vi "New Durability Tank Cal UI.vi"(11 "Calling VI Ref":refnum<vi>) -> ()   [LabVIEW 2019]
uses:
  Type Defs/Units Type Def (DAQ Rack).ctl
  Type Defs/New Channel Type Def (RIO).ctl
  Type Defs/Targets Type Def.ctl
  Type Defs/Target Cluster Type Def.ctl
  Type Defs/Setpoint Cluster Type Def.ctl
  Type Defs/Rack Version Type Def.ctl
  Type Defs/Registered System.ctl
  Type Defs/System Type.ctl
  Type Defs/TCP Data Stream Mode (PC).ctl
  <vilib>/Utility/miscctls.llb/LVRowAndColumnTypeDef.ctl
  <vilib>/Utility/file.llb/Write To Spreadsheet File (string).vi
  <vilib>/Utility/file.llb/Read From Spreadsheet File (string).vi
  <userlib>/_OpenG.lib/array/array.llb/Remove Duplicates from 1D Array (DBL)__ogtk.vi
  <userlib>/_OpenG.lib/array/array.llb/Search 1D Array (String)__ogtk.vi
  <vilib>/ptbypt/NI_PtbyPt.lvlib
  <vilib>/Analysis/NI_AALPro.lvlib
  <resource>/objmgr/daqmx.rc
  <vilib>/Utility/config.llb/NI_LVConfig.lvlib
  <vilib>/FTP/NI_FTP.lvlib
panel:
  out "RIO Found":bool
  out "Lost Connection":bool
  in  "Stop Second Loop":bool
  out "a0":dbl format="%#.4g"
  out "a2":dbl format="%#.4g"
  out "a1":dbl format="%#.4g"
  out "a3":dbl format="%#.4g"
  out "a4":dbl format="%#.4g"
  in  "App Dir":path
  in  "Load Indicator Tab":enum32{"Page 1"}(tab)
  in  "Header Tab":enum32{"Page 1", "Page 2"}(tab)
  in  "Header OK":bool
  in  "Header Cancel":bool
  in  "Header Comments":string[][](table)=[[""], [""], [""]]
  in  "Cal Standards Table":string[][](table)=[["", ""], ["", ""], ["", ""], ["", ""], ["", ""]]
  in  "Sys Cal Table":string[][](table)=[["", ""], ["", ""], ["", ""], ["", ""], ["", ""]]
  in  "Header Table 1":string[][](table)=[[""], [""], [""], [""], [""], [""], [""], [""]]
  in  "Header Table 2":string[][](table)=[[""], [""], [""], [""], [""], [""], [""]]
  in  "debug":bool=TRUE
  in  "Output Tab":enum32{"Page 1", "Page 2"}(tab)
  out "Row":i32
  in  "Main Tab":enum32{"Page 1", "Page 2"}(tab)
  in  "Transfer Cal":bool
  in  "Verify Tab":enum32{"Page 1", "Page 2"}(tab)
  out "Ver Reading":dbl=0.0016 caption="reading" format="%#.4g"
  in  "Hide Devs":bool
  in  "Auto":bool
  in  "Hide Cal Values":bool
  in  "Verify Edit":bool
  in  "Verify Table":string[][](table)=[["", "0", "0"], ["", "3", "3"], ["", "6", "6"], ["", "9", "9"], ["", "12", "12"], ["", "15", "15"], ["", "", ""], ["", "", ""], ["", "", ""], ["", "", ""]]
  in  "Verify Read":bool
  in  "ms":u32=1000
  in  "avg":i32=5
  in  "Save Cal":bool
  in  "Cancel Verify":bool
  in  "Cal Tab":enum32{"Apply", "Cal"}(tab)
  in  "Cancel Cal":bool
  in  "Apply Cal":bool
  in  "Confirm Cal Point":bool
  in  "Master Value":dbl caption="cal pt" format="%#.4g"
  out "Cal Reading":dbl=0.0016 caption="reading" format="%#.4g"
  in  "Channel to Cal":T1
  in  "4th Point Cal":bool
  out "Reading Value 4":dbl caption="reading" format="%#.4g"
  in  "Cal Value 4":dbl caption="cal pt" format="%#.4g"
  in  "5th Point Cal":bool
  out "Reading Value 5":dbl caption="reading" format="%#.4g"
  in  "Cal Value 5":dbl caption="cal pt" format="%#.4g"
  in  "Start Verification":bool
  in  "Header":bool
  out "Cal Table":string[][](table)=[["AI-00", "V", "", "", "", "", "", "", "", "", "", "", "", "", "", "", "", "", "", "", "", "", "", "", "", "", "", "", "", "", "", ""], ["AI-01", "V", "", "", "", "", "", "", "", "", "", "", "", "", "", "", "", "", "", "", "", "", "", "", "", "", "", "", "", "", "", ""], ["AI-02", "V", "", "", "", "", "", "", "", "", "", "", "", "", "", "", "", "", "", "", "", "", "", "", "", "", "", "", "", "", "", ""], ["AI-03", "V", "", "", "", "", "", "", "", "", "", "", "", "", "", "", "", "", "", "", "", "", "", "", "", "", "", "", "", "", "", ""], ["AI-04", "V", "", "", "", "", "", "", "", "", "", "", "", "", "", "", "", "", "", "", "", "", "", "", "", "", "", "", "", "", "", ""], ["AI-05", "V", "", "", "", "", "", "", "", "", "", "", "", "", "", "", "", "", "", "", "", "", "", "", "", "", "", "", "", "", "", ""], ["AI-06", "V", "", "", "", "", "", "", "", "", "", "", "", "", "", "", "", "", "", "", "", "", "", "", "", "", "", "", "", "", "", ""], ["AI-07", "V", "", "", "", "", "", "", "", "", "", "", "", "", "", "", "", "", "", "", "", "", "", "", "", "", "", "", "", "", "", ""], ["AI-08", "V", "", "", "", "", "", "", "", "", "", "", "", "", "", "", "", "", "", "", "", "", "", "", "", "", "", "", "", "", "", ""], ["AI-09", "V", "", "", "", "", "", "", "", "", "", "", "", "", "", "", "", "", "", "", "", "", "", "", "", "", "", "", "", "", "", ""], ["AI-10", "V", "", "", "", "", "", "", "", "", "", "", "", "", "", "", "", "", "", "", "", "", "", "", "", "", "", "", "", "", "", ""], ["AI-11", "V", "", "", "", "", "", "", "", "", "", "", "", "", "", "", "", "", "", "", "", "", "", "", "", "", "", "", "", "", "", ""], ["AI-12", "V", "", "", "", "", "", "", "", "", "", "", "", "", "", "", "", "", "", "", "", "", "", "", "", "", "", "", "", "", "", ""], ["AI-13", "V", "", "", "", "", "", "", "", "", "", "", "", "", "", "", "", "", "", "", "", "", "", "", "", "", "", "", "", "", "", ""], ["AI-14", "V", "", "", "", "", "", "", "", "", "", "", "", "", "", "", "", "", "", "", "", "", "", "", "", "", "", "", "", "", "", ""], ["AI-15", "V", "", "", "", "", "", "", "", "", "", "", "", "", "", "", "", "", "", "", "", "", "", "", "", "", "", "", "", "", "", ""], ["AI-16", "V", "", "", "", "", "", "", "", "", "", "", "", "", "", "", "", "", "", "", "", "", "", "", "", "", "", "", "", "", "", ""], ["AI-17", "V", "", "", "", "", "", "", "", "", "", "", "", "", "", "", "", "", "", "", "", "", "", "", "", "", "", "", "", "", "", ""], ["AI-18", "V", "", "", "", "", "", "", "", "", "", "", "", "", "", "", "", "", "", "", "", "", "", "", "", "", "", "", "", "", "", ""], ["AI-19", "V", "", "", "", "", "", "", "", "", "", "", "", "", "", "", "", "", "", "", "", "", "", "", "", "", "", "", "", "", "", ""], ["AI-20", "V", "", "", "", "", "", "", "", "", "", "", "", "", "", "", "", "", "", "", "", "", "", "", "", "", "", "", "", "", "", ""], ["AI-21", "V", "", "", "", "", "", "", "", "", "", "", "", "", "", "", "", "", "", "", "", "", "", "", "", "", "", "", "", "", "", ""], ["AI-22", "V", "", "", "", "", "", "", "", "", "", "", "", "", "", "", "", "", "", "", "", "", "", "", "", "", "", "", "", "", "", ""], ["AI-23", "V", "", "", "", "", "", "", "", "", "", "", "", "", "", "", "", "", "", "", "", "", "", "", "", "", "", "", "", "", "", ""], ["AI-24", "V", "", "", "", "", "", "", "", "", "", "", "", "", "", "", "", "", "", "", "", "", "", "", "", "", "", "", "", "", "", ""], ["AI-25", "V", "", "", "", "", "", "", "", "", "", "", "", "", "", "", "", "", "", "", "", "", "", "", "", "", "", "", "", "", "", ""], ["AI-26", "V", "", "", "", "", "", "", "", "", "", "", "", "", "", "", "", "", "", "", "", "", "", "", "", "", "", "", "", "", "", ""], ["AI-27", "V", "", "", "", "", "", "", "", "", "", "", "", "", "", "", "", "", "", "", "", "", "", "", "", "", "", "", "", "", "", ""], ["AI-28", "V", "", "", "", "", "", "", "", "", "", "", "", "", "", "", "", "", "", "", "", "", "", "", "", "", "", "", "", "", "", ""], ["AI-29", "V", "", "", "", "", "", "", "", "", "", "", "", "", "", "", "", "", "", "", "", "", "", "", "", "", "", "", "", "", "", ""], ["AI-30", "V", "", "", "", "", "", "", "", "", "", "", "", "", "", "", "", "", "", "", "", "", "", "", "", "", "", "", "", "", "", ""], ["AI-31", "V", "", "", "", "", "", "", "", "", "", "", "", "", "", "", "", "", "", "", "", "", "", "", "", "", "", "", "", "", "", ""], ["TC-00", "degF", "", "", "", "", "", "", "", "", "", "", "", "", "", "", "", "", "", "", "", "", "", "", "", "", "", "", "", "", "", ""], ["TC-01", "degF", "", "", "", "", "", "", "", "", "", "", "", "", "", "", "", "", "", "", "", "", "", "", "", "", "", "", "", "", "", ""], ["TC-02", "degF", "", "", "", "", "", "", "", "", "", "", "", "", "", "", "", "", "", "", "", "", "", "", "", "", "", "", "", "", "", ""], ["TC-03", "degF", "", "", "", "", "", "", "", "", "", "", "", "", "", "", "", "", "", "", "", "", "", "", "", "", "", "", "", "", "", ""], ["TC-04", "degF", "", "", "", "", "", "", "", "", "", "", "", "", "", "", "", "", "", "", "", "", "", "", "", "", "", "", "", "", "", ""], ["TC-05", "degF", "", "", "", "", "", "", "", "", "", "", "", "", "", "", "", "", "", "", "", "", "", "", "", "", "", "", "", "", "", ""], ["TC-06", "degF", "", "", "", "", "", "", "", "", "", "", "", "", "", "", "", "", "", "", "", "", "", "", "", "", "", "", "", "", "", ""], ["TC-07", "degF", "", "", "", "", "", "", "", "", "", "", "", "", "", "", "", "", "", "", "", "", "", "", "", "", "", "", "", "", "", ""], ["TC-08", "degF", "", "", "", "", "", "", "", "", "", "", "", "", "", "", "", "", "", "", "", "", "", "", "", "", "", "", "", "", "", ""], ["TC-09", "degF", "", "", "", "", "", "", "", "", "", "", "", "", "", "", "", "", "", "", "", "", "", "", "", "", "", "", "", "", "", ""], ["TC-10", "degF", "", "", "", "", "", "", "", "", "", "", "", "", "", "", "", "", "", "", "", "", "", "", "", "", "", "", "", "", "", ""], ["TC-11", "degF", "", "", "", "", "", "", "", "", "", "", "", "", "", "", "", "", "", "", "", "", "", "", "", "", "", "", "", "", "", ""], ["TC-12", "degF", "", "", "", "", "", "", "", "", "", "", "", "", "", "", "", "", "", "", "", "", "", "", "", "", "", "", "", "", "", ""], ["TC-13", "degF", "", "", "", "", "", "", "", "", "", "", "", "", "", "", "", "", "", "", "", "", "", "", "", "", "", "", "", "", "", ""], ["TC-14", "degF", "", "", "", "", "", "", "", "", "", "", "", "", "", "", "", "", "", "", "", "", "", "", "", "", "", "", "", "", "", ""], ["TC-15", "degF", "", "", "", "", "", "", "", "", "", "", "", "", "", "", "", "", "", "", "", "", "", "", "", "", "", "", "", "", "", ""], ["", "", "", "", "", "", "", "", "", "", "", "", "", "", "", "", "", "", "", "", "", "", "", "", "", "", "", "", "", "", "", ""]]
  out "Tank IP:":string
  in  "Start Cal":bool
  in  "1st Point Cal":bool
  out "Reading Value 1":dbl caption="Read Data" format="%#.4g"
  in  "Cal Value 1":dbl caption="Cal Point" format="%#.4g"
  in  "2nd Point Cal":bool
  out "Reading Value 2":dbl caption="reading" format="%#.4g"
  in  "Cal Value 2":dbl caption="cal pt" format="%#.4g"
  in  "Cal Unit":T2
  in  "3rd Point Cal":bool
  out "Reading Value 3":dbl caption="reading" format="%#.4g"
  in  "Cal Value 3":dbl caption="cal pt" format="%#.4g"
  in  "View Spreadsheet":bool
  # "Channel Data"
  # "System Calibration Components"
  # "Calibration Standards Used"
  # "Output Control"
  # "Enter Header Info"
  # "Calibration"
  # "Verification"
  # "Select Channel to Calibrate"
  # "Cal Spreadsheet"
  # "*Excel must be closed to return control to this app."
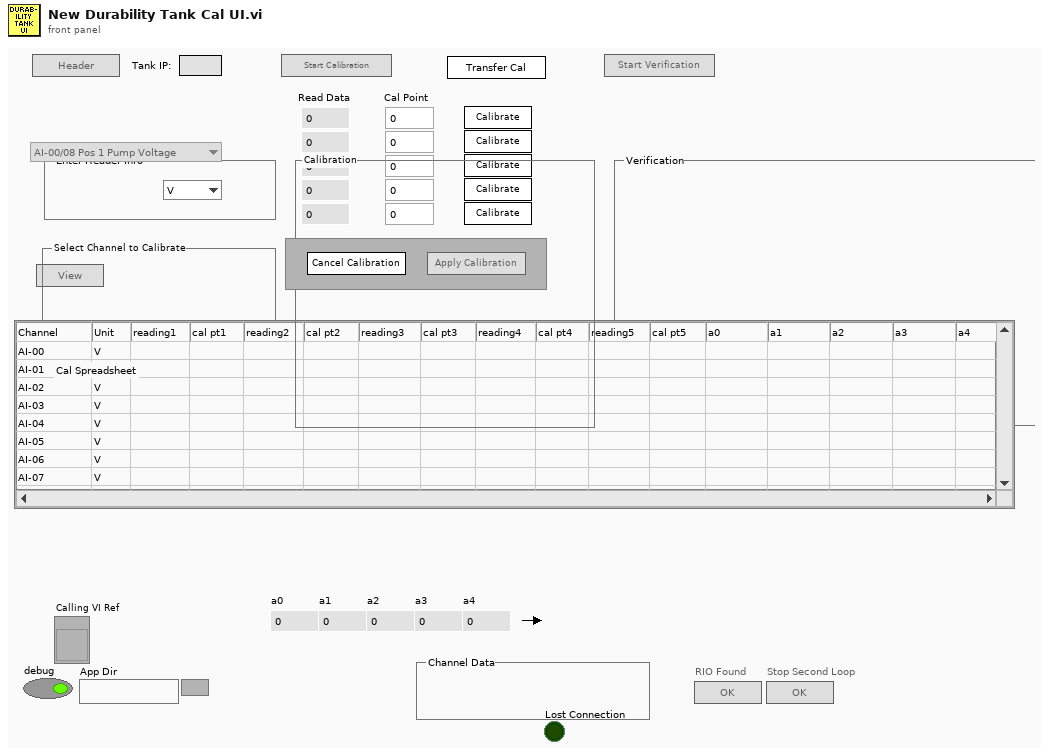
[diagram p1: front panel]
types:
  T1 = typedef "New Channel Type Def (RIO).ctl" = enum16{"AI-00/08 Pos 1 Pump Voltage", "AI-01/09 Pos 2 Pump Voltage", "AI-02/10 Pos 3 Pump Voltage", "AI-03/11 Pos 4 Pump Voltage", "AI-04/12 Pos 5 Pump Voltage", "AI-05/13 Pos 6 Pump Voltage", "AI-06 Spare", "AI-14 Spare", "AI-07 Spare", "AI-15 Power Supply Voltage", "AI-16 Pos 1 Pump Current", "AI-17 Pos 2 Pump Current", "AI-18 Pos 3 Pump Current", "AI-19 Pos 4 Pump Current", "AI-20 Pos 5 Pump Current", "AI-21 Pos 6 Pump Current", "AI-16 Pos 1 Pump Speed", "AI-17 Pos 2 Pump Speed", "AI-18 Pos 3 Pump Speed", "AI-19 Pos 4 Pump Speed", "AI-20 Pos 5 Pump Speed", "AI-21 Pos 6 Pump Speed", "AI-22 Pos 1 Controller Current", "AI-23 Pos 2 Controller Current", "AI-24 Pos 3 Controller Current", "AI-25 Pos 4 Controller Current", "AI-26 Pos 5 Controller Current", "AI-27 Pos 6 Controller Current", "AI-28 Tank 1 Temperature", "AI-29 Tank 2 Temperature", "AI-30 Pos 1 Pump Pressure", "AI-31 Pos 2 Pump Pressure", "AI-32 Pos 3 Pump Pressure", "AI-33 Pos 4 Pump Pressure", "AI-34 Pos 5 Pump Pressure", "AI-35 Pos 6 Pump Pressure", "AI-36 Pos 1 Pump Flow", "AI-37 Pos 2 Pump Flow", "AI-38 Pos 3 Pump Flow", "AI-39 Pos 4 Pump Flow", "AI-40 Pos 5 Pump Flow", "AI-41 Pos 6 Pump Flow", "AI-42 Spare", "AI-43 Spare", "AI-44 Spare", "AI-45 Spare", "AI-46 Spare", "AI-47 Spare", "AI-00/08 Pos 1 Controller Voltage", "AI-01/09 Pos 2 Controller Voltage", "AI-02/10 Pos 3 Controller Voltage", "AI-03/11 Pos 4 Controller Voltage", "AI-04/12 Pos 5 Controller Voltage", "AI-05/13 Pos 6 Controller Voltage"}
  T2 = typedef "Units Type Def (DAQ Rack).ctl" = enum16{"V", "mA", "A", "Hz", "deg C"}
  T3 = typedef "Registered System.ctl" = cluster{"System Type":T4, "Serial Number":u32, "ID":string, "Cal File?":bool}
  T4 = typedef "System Type.ctl" = enum16{"DAQ Rack", "DAQ Cart", "RIO", "unknown", "open"}
  T5 = typedef "Rack Version Type Def.ctl" = enum16{"Volts & TC", "Volts", "RIO", "Volts & Current", "Cart"}
  T6 = typedef "Targets Type Def.ctl" = cluster{"V Targets":T7, "5V Targets":T7, "mA Targets":T7, "A Targets":T7, "Hz Targets":T7, "TC Targets":T7, "V Setpoints":T8, "5V Setpoints":T8, "mA Setpoints ":T8, "A Setpoints":T8, "Hz Setpoints":T8, "25A Setpoints":T8, "25A Targets":T7, "CT Targets":T7, "DegC Targets":T7, "kPa Targets":T7, "LpH Targets":T7, "CT Setpoints":T8, "DegC Setpoints":T8, "kPa Setpoints":T8, "LpH Setpoints":T8}
  T7 = typedef "Target Cluster Type Def.ctl" = cluster{"target1":dbl, "target2":dbl, "target3":dbl, "target4":dbl, "target5":dbl, "target6":dbl, "target7":dbl, "target8":dbl, "target9":dbl, "target10":dbl}
  T8 = typedef "Setpoint Cluster Type Def.ctl" = cluster{"setpoint1":dbl, "setpoint2":dbl, "setpoint3":dbl, "setpoint4":dbl, "setpoint5":dbl}
  T9 = cluster{"Error":errorcluster, "Cal Log":string[][], "Cal Log Header":string[], "Cal Files Base Path":path, "Default Cal Log":string[][], "Samples to Avg":i32, "Base Path":path, "Cal Targets Path":path, "Calling VI Ref":refnum<vi>, "Selected Chassis":tag, "debug":bool, "Verify Table":string[][], "Cal Template Path":path, "Cal Spreadsheet Path":path, "Verify Table Ref":refnum<vi>, "Init Mean":bool, "Auto":bool, "App Dir":path, "DAQ Rack":string, "Cal File Path":path, "Targets":T6, "Cal Unit":T2, "Channel to Cal":T1, "Rack Version":T5, "Verification":bool, "Registered Systems":T3[], "Desired System":T3, "Cal Target Array":string[], "LastCalPt":i32, "StreamCtrlActive":bool}
  T10 = enum8{"Enabled", "Disabled", "Disabled and Grayed Out"}
  T11 = typedef "TCP Data Stream Mode (PC).ctl" = enum16{"Init", "Read Data", "Close"}
  T12 = typedef "LVRowAndColumnTypeDef.ctl" = cluster{"Row":i32, "Column":i32}
  T13 = enum32{"Bad", "Idle", "Run top level", "Running"}
  T14 = cluster{"[0]":dbl, "[1]":dbl, "[2]":dbl, "[3]":dbl, "[4]":dbl, "[5]":dbl, "[6]":dbl, "[7]":dbl, "[8]":dbl, "[9]":dbl}
  T15 = typedef "NI_LVConfig.lvlib/Config Data RefNum.ctl" = refnum<k1>
  T16 = cluster{"Error":errorcluster, "Cal Log":string[][], "Cal Log Header":string[], "Cal Files Base Path":path, "Default Cal Log":string[][], "Samples to Avg":i32, "Base Path":path, "Cal Targets Path":path, "Calling VI Ref":refnum<vi>, "Selected Chassis":tag, "debug":bool, "Verify Table":string[][], "Cal Template Path":path, "Cal Spreadsheet Path":path, "Verify Table Ref":refnum<vi>, "Init Mean":bool, "Auto":bool, "App Dir":path, "DAQ Rack":string, "Cal File Path":path, "Targets":T6, "Cal Unit":T2, "Channel to Cal":T1, "Rack Version":T5, "Verification":bool, "Registered Systems":T3[], "Desired System":T3, "Cal Target Array":string[], "LastCalPt":i32}
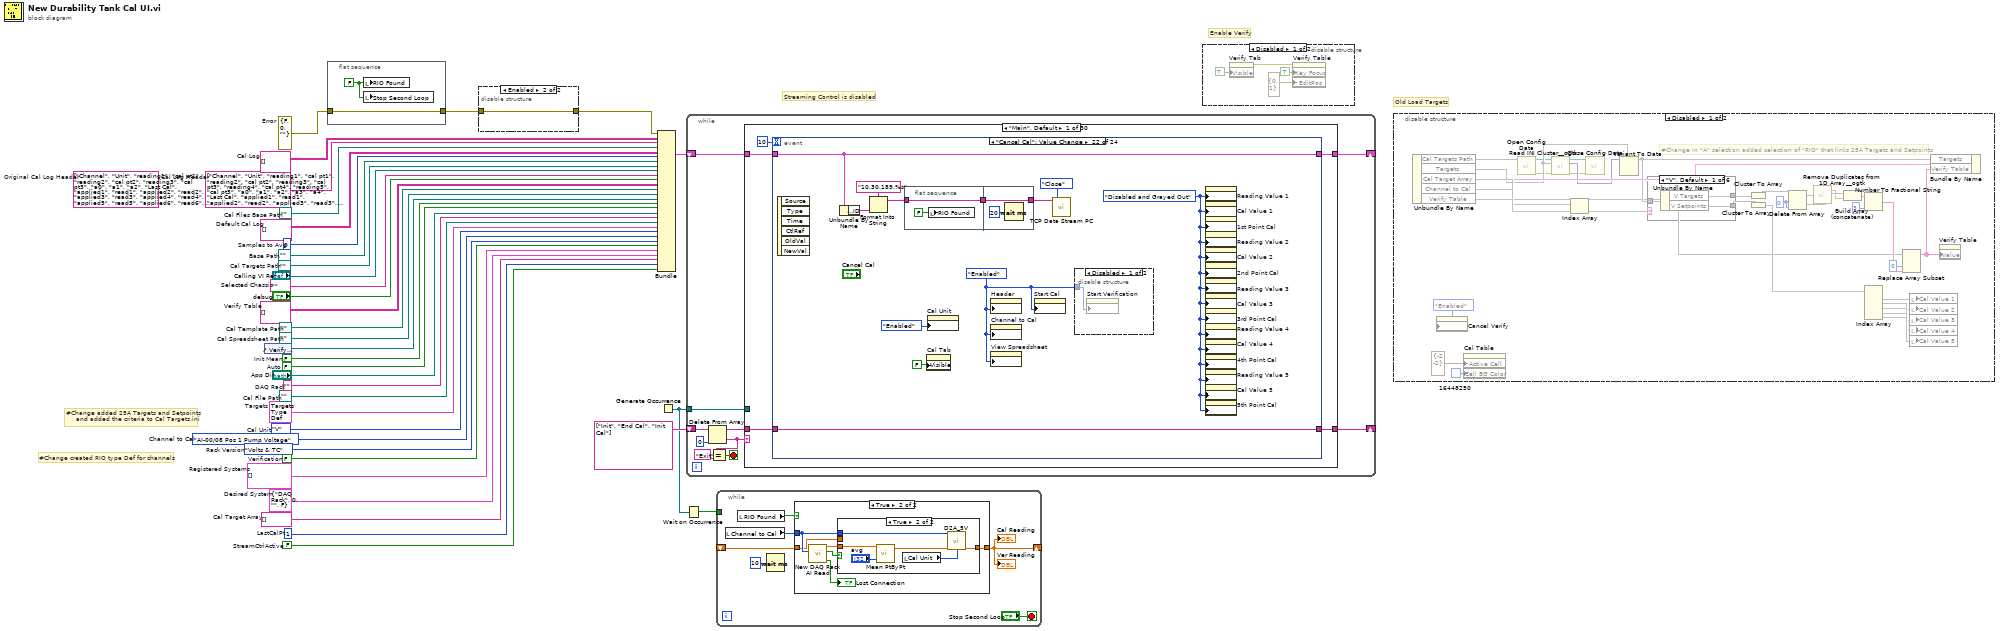
[diagram p0: block diagram]
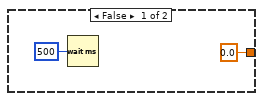
[diagram p2: hidden frame]
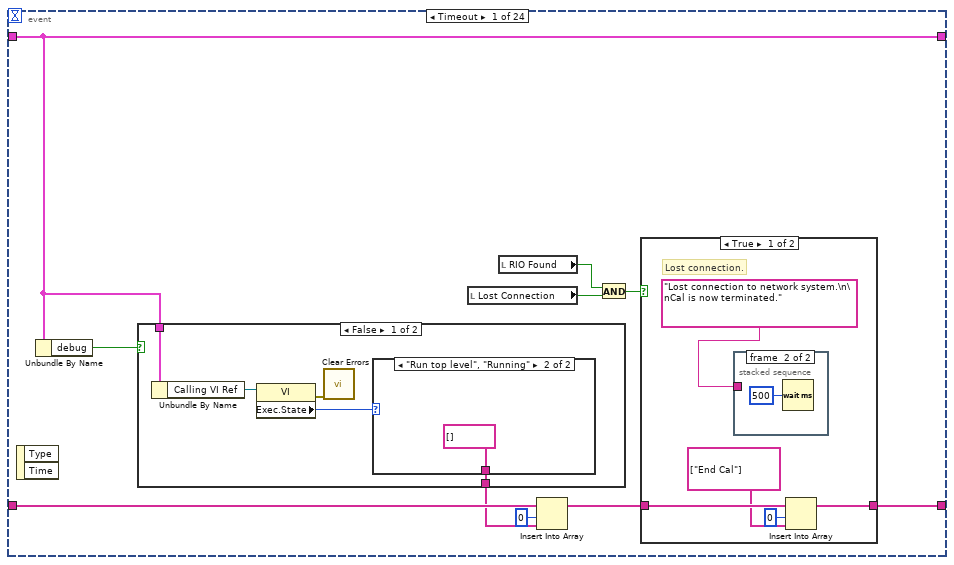
[diagram p4: hidden frame]
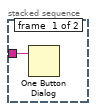
[diagram p5: hidden frame]
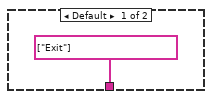
[diagram p7: hidden frame]
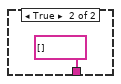
[diagram p8: hidden frame]
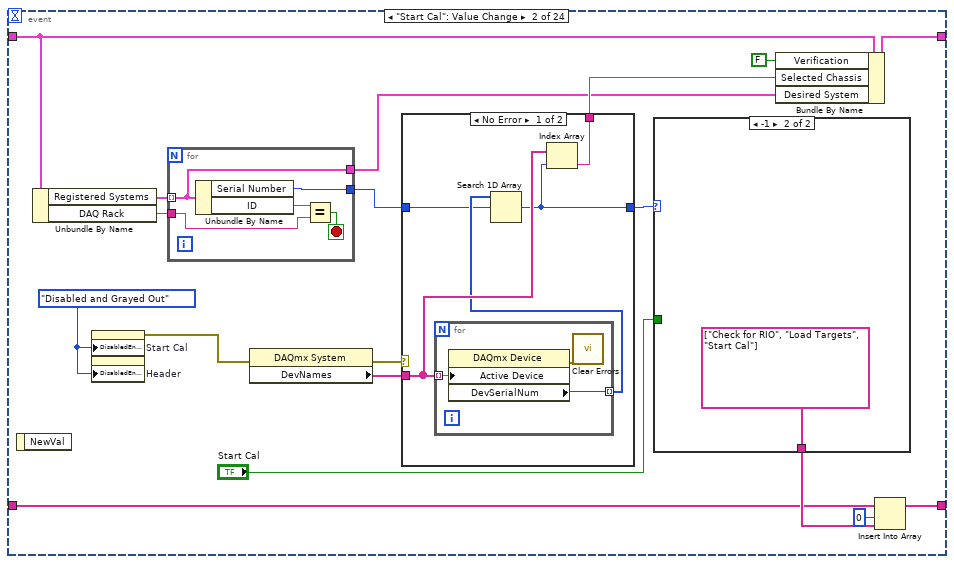
[diagram p9: hidden frame]
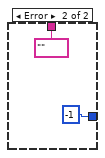
[diagram p10: hidden frame]
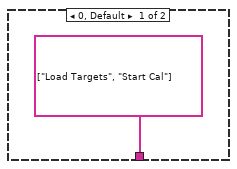
[diagram p11: hidden frame]
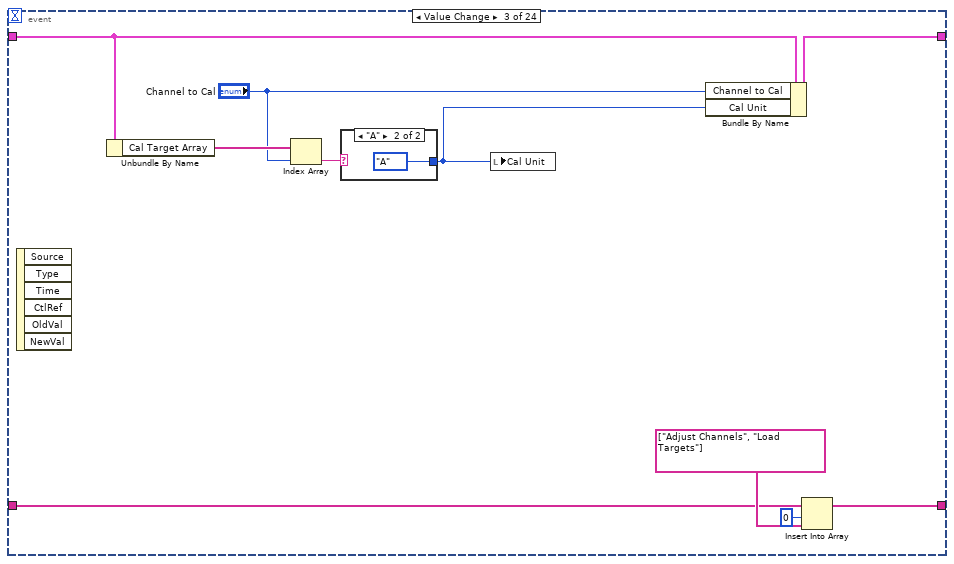
[diagram p12: hidden frame]
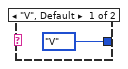
[diagram p13: hidden frame]
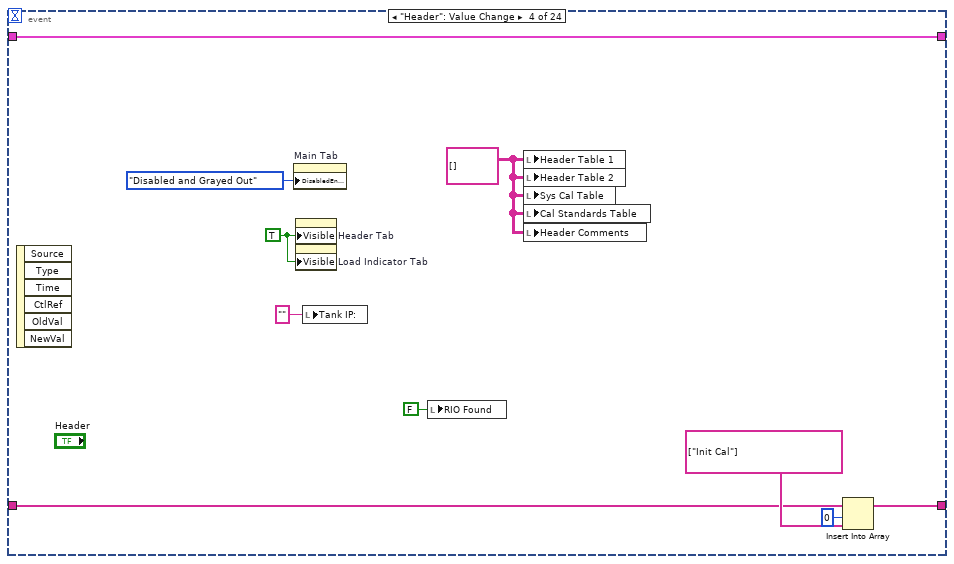
[diagram p14: hidden frame]
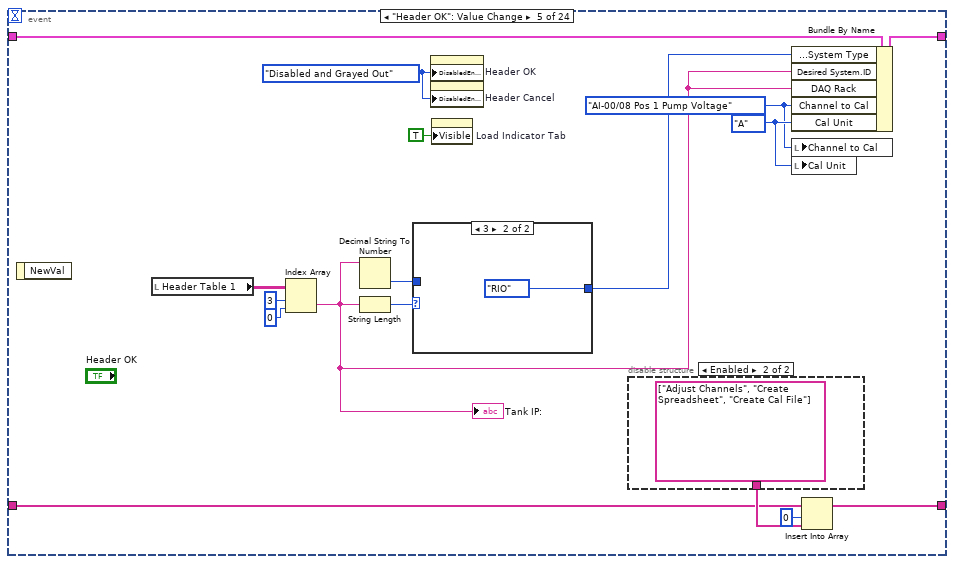
[diagram p15: hidden frame]
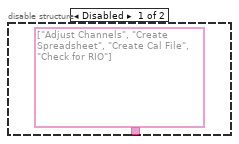
[diagram p16: hidden frame]
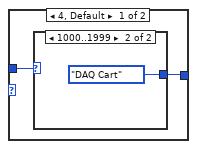
[diagram p17: hidden frame]
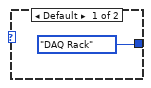
[diagram p18: hidden frame]
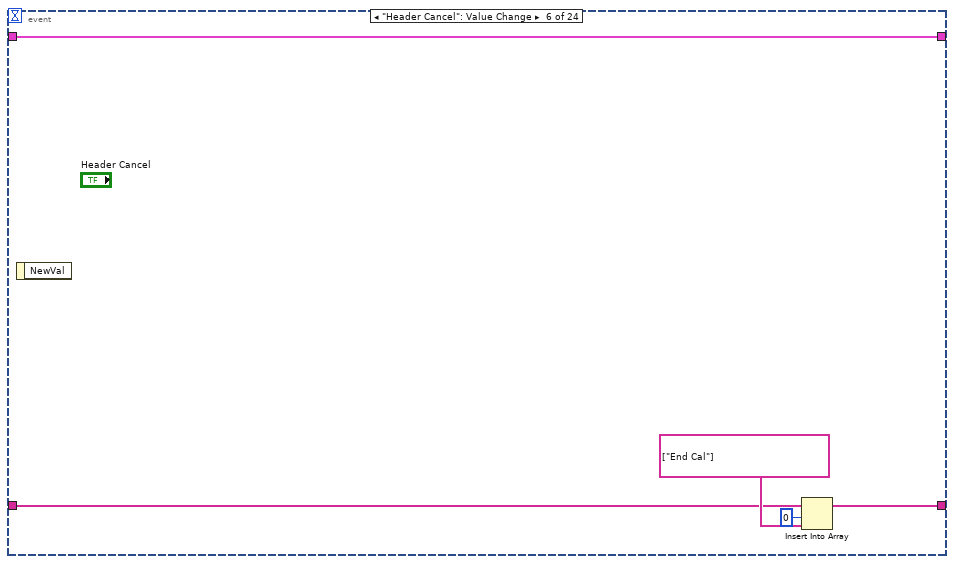
[diagram p19: hidden frame]
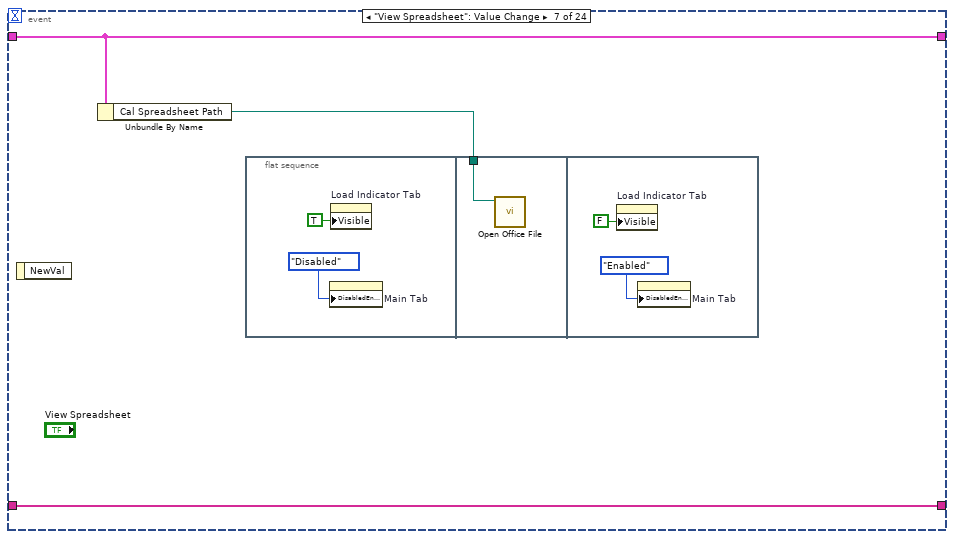
[diagram p20: hidden frame]
diagram:
  w7 = FALSE  # StreamCtrlActive
  w8 = 1  # LastCalPt
  w10 = New_Channel_Type_Def_(RIO)."AI-00/08 Pos 1 Pump Voltage"  # Channel to Cal
  w11 = string[] ["Channel", "Unit", "reading1", "cal pt1", "reading2", "cal pt2", "reading3", "cal pt3", "reading4", "cal pt4", "reading5", "cal pt5", "a0", "a1", "a2", "a3", "a4", "Last Cal", "applied1", "read1", "applied2", "read2", "applied3", "read3", "applied4", "read4", "applied5", "read5", "applied6", "read6", "applied7", "read7", "applied8", "read8", "applied9", "read9", "applied10", "read10"]  # Cal Log Header
  w12 = string[] []  # Cal Target Array
  w13 = T3 {"System Type"=enum."DAQ Rack", "Serial Number"=0, "ID"="", "Cal File?"=FALSE}  # Desired System
  w14 = T3[] []  # Registered Systems
  w15 = FALSE  # Verification
  w16 = Rack_Version_Type_Def."Volts & TC"  # Rack Version
  w17 = Units_Type_Def_(DAQ_Rack)."V"  # Cal Unit
  w18 = T6 {"V Targets"={"target1"=0.0, "target2"=0.0, "target3"=0.0, "target4"=0.0, "target5"=0.0, "target6"=0.0, "target7"=0.0, "target8"=0.0, "target9"=0.0, "target10"=0.0}, "5V Targets"={"target1"=0.0, "target2"=0.0, "target3"=0.0, "target4"=0.0, "target5"=0.0, "target6"=0.0, "target7"=0.0, "target8"=0.0, "target9"=0.0, "target10"=0.0}, "mA Targets"={"target1"=0.0, "target2"=0.0, "target3"=0.0, "target4"=0.0, "target5"=0.0, "target6"=0.0, "target7"=0.0, "target8"=0.0, "target9"=1.0, "target10"=0.0}, "A Targets"={"target1"=0.0, "target2"=0.0, "target3"=0.0, "target4"=0.0, "target5"=0.0, "target6"=0.0, "target7"=0.0, "target8"=0.0, "target9"=0.0, "target10"=0.0}, "Hz Targets"={"target1"=0.0, "target2"=0.0, "target3"=0.0, "target4"=0.0, "target5"=0.0, "target6"=0.0, "target7"=0.0, "target8"=0.0, "target9"=0.0, "target10"=0.0}, "TC Targets"={"target1"=0.0, "target2"=0.0, "target3"=0.0, "target4"=0.0, "target5"=0.0, "target6"=0.0, "target7"=0.0, "target8"=0.0, "target9"=0.0, "target10"=0.0}, "V Setpoints"={"setpoint1"=0.0, "setpoint2"=0.0, "setpoint3"=0.0, "setpoint4"=0.0, "setpoint5"=0.0}, "5V Setpoints"={"setpoint1"=0.0, "setpoint2"=0.0, "setpoint3"=0.0, "setpoint4"=0.0, "setpoint5"=0.0}, "mA Setpoints "={"setpoint1"=0.0, "setpoint2"=0.0, "setpoint3"=0.0, "setpoint4"=0.0, "setpoint5"=0.0}, "A Setpoints"={"setpoint1"=0.0, "setpoint2"=0.0, "setpoint3"=0.0, "setpoint4"=0.0, "setpoint5"=0.0}, "Hz Setpoints"={"setpoint1"=0.0, "setpoint2"=0.0, "setpoint3"=0.0, "setpoint4"=0.0, "setpoint5"=0.0}, "25A Setpoints"={"setpoint1"=0.0, "setpoint2"=0.0, "setpoint3"=0.0, "setpoint4"=0.0, "setpoint5"=0.0}, "25A Targets"={"target1"=0.0, "target2"=0.0, "target3"=0.0, "target4"=0.0, "target5"=0.0, "target6"=0.0, "target7"=0.0, "target8"=0.0, "target9"=0.0, "target10"=0.0}, "CT Targets"={"target1"=0.0, "target2"=0.0, "target3"=0.0, "target4"=0.0, "target5"=0.0, "target6"=0.0, "target7"=0.0, "target8"=0.0, "target9"=0.0, "target10"=0.0}, "DegC Targets"={"target1"=0.0, "target2"=0.0, "target3"=0.0, "target4"=0.0, "target5"=0.0, "target6"=0.0, "target7"=0.0, "target8"=0.0, "target9"=0.0, "target10"=0.0}, "kPa Targets"={"target1"=0.0, "target2"=0.0, "target3"=0.0, "target4"=0.0, "target5"=0.0, "target6"=0.0, "target7"=0.0, "target8"=0.0, "target9"=0.0, "target10"=0.0}, "LpH Targets"={"target1"=0.0, "target2"=0.0, "target3"=0.0, "target4"=0.0, "target5"=0.0, "target6"=0.0, "target7"=0.0, "target8"=0.0, "target9"=0.0, "target10"=0.0}, "CT Setpoints"={"setpoint1"=0.0, "setpoint2"=0.0, "setpoint3"=0.0, "setpoint4"=0.0, "setpoint5"=0.0}, "DegC Setpoints"={"setpoint1"=0.0, "setpoint2"=0.0, "setpoint3"=0.0, "setpoint4"=0.0, "setpoint5"=0.0}, "kPa Setpoints"={"setpoint1"=0.0, "setpoint2"=0.0, "setpoint3"=0.0, "setpoint4"=0.0, "setpoint5"=0.0}, "LpH Setpoints"={"setpoint1"=0.0, "setpoint2"=0.0, "setpoint3"=0.0, "setpoint4"=0.0, "setpoint5"=0.0}}  # Targets
  w19 = path ""  # Cal File Path
  w20 = ""  # DAQ Rack
  w22 = FALSE  # Auto
  w23 = FALSE  # Init Mean
  w25 = path ""  # Cal Spreadsheet Path
  w26 = path ""  # Cal Template Path
  w27 = string[][] []  # Verify Table
  w29 = tag ""  # Selected Chassis
  w31 = path ""  # Cal Targets Path
  w32 = path ""  # Base Path
  w33 = 0  # Samples to Avg
  w34 = string[][] []  # Default Cal Log
  w35 = path ""  # Cal Files Base Path
  (unwired) string[] ["Channel", "Unit", "reading1", "cal pt1", "reading2", "cal pt2", "reading3", "cal pt3", "a0", "a1", "a2", "Last Cal", "applied1", "read1", "applied2", "read2", "applied3", "read3", "applied4", "read4", "applied5", "read5", "applied6", "read6", "applied7", "read7", "applied8", "read8", "applied9", "read9", "applied10", "read10"]  # Original Cal Log Header
  w36 = string[][] []  # Cal Log
  w9 = errorcluster {"status"=FALSE, "code"=0, "source"=""}  # Error
  # "Old Load Targets"
  # "Streaming Control is disabled"
  # "Enable Verify"
  # "#Change created RIO type Def for channels"
  # "#Change added 25A Targets and Setpoints\n     and added the criteria to Cal Targets.ini"
  n1 = control-ref of="Verify Table Ref"() -> (w24:refnum<vi>)
  n2 = flat-sequence {
    tunnel: w9 -> [w38]
    tunnel: [w38] -> w6
    frame #0 {
      w37 = FALSE ("RIO Found")
      n3 = local write "RIO Found"(w37) -> ()
      n4 = local write "Stop Second Loop"(w37) -> ()
    }
  }
  n5 = disable-structure shown="Enabled" {
    disable-tunnel: w6 -> [w42 w43]
    disable-tunnel: [w40 w43] -> w5
    frame Disabled {
      w39 = TRUE ("Visible")
      n6 = property on="Cal Tab" class="TabCtl (strict)"(error in=w42, "Visible"=w39) -> (error out=w41:errorcluster)  [unwired: 1 in, 1 out]
      n7 = property on="Verify Tab" class="TabCtl (strict)"(error in=w41, "Visible"=w39) -> (error out=w40:errorcluster)  [unwired: 1 in, 1 out]
    }
    frame Enabled {
    }
  }
  n8 = Bundle("Error"=w5, "Cal Log"=w36, "Cal Log Header"=w11, "Cal Files Base Path"=w35, "Default Cal Log"=w34, "Samples to Avg"=w33, "Base Path"=w32, "Cal Targets Path"=w31, "Calling VI Ref"="Calling VI Ref", "Selected Chassis"=w29, "debug"="debug", "Verify Table"=w27, "Cal Template Path"=w26, "Cal Spreadsheet Path"=w25, "Verify Table Ref"=w24, "Init Mean"=w23, "Auto"=w22, "App Dir"="App Dir", "DAQ Rack"=w20, "Cal File Path"=w19, "Targets"=w18, "Cal Unit"=w17, "Channel to Cal"=w10, "Rack Version"=w16, "Verification"=w15, "Registered Systems"=w14, "Desired System"=w13, "Cal Target Array"=w12, "LastCalPt"=w8, "StreamCtrlActive"=w7) -> (w3:T9)  [unwired: 1 in]
  n9 = Generate Occurrence() -> (w2:refnum<k4>)
  n10 = Wait on Occurrence(2:w2) -> (0:w1:bool)  [unwired: 2 in]
  n11 = while {
    shift-right: [w46] -> _
    shift-left: string[] ["Init", "End Cal", "Init Cal"] -> [w53]
    shift-right: [w48] -> _
    shift-left: w3 -> [w49]
    tunnel: w2 -> [w44]
    stop <- w52 stop-if-true
    n12 = Delete From Array(array=w53, index=0) -> (deleted portion=w45:string, array with subset deleted=w51:string[])  [unwired: 1 in]
    n13 = Equal?(x=w45, y="Exit" ("x")) -> (x = y?=w52:bool)
    n14 = case shown="\"Main\", Default" w45 {
      selector: w45 -> [_ _ _ _ _ _ _ _ _ _ _ _ _ _ _ w851 _ _ _ _ _ _ _ _ _ _ _ _ _ _]
      tunnel: w51 -> [w57 w425 w440 w448 w464 w513 w543 w546 w550 w581 w610 w639 w663 w721 w840 w853 w867 w883 w967 w994 w1004 w1067 w1145 w1168 w1185 w1196 w1219 w1232 w1240 w1243]
      tunnel: w49 -> [w56 w418 w441 w454 w461 w512 w542 w545 w548 w584 w612 w633 w661 w769 w844 w848 w868 w877 w953 w978 w1005 w1028 w1106 w1167 w1183 w1194 w1216 w1229 w1238 w1242]
      tunnel: [w55 w400 w441 w453 w461 w511 w541 w545 w548 w583 w612 w632 w665 w778 w844 w847 w868 w877 w953 w973 w1005 w1028 w1106 w1167 w1182 w1194 w1216 w1229 w1239 w1242] -> w48
      tunnel: [w54 w425 w440 w445 w463 w513 w543 w546 w549 w582 w611 w640 w664 w720 w840 w853 w867 w884 w966 w995 w1004 w1068 w1146 w1168 w1184 w1195 w1219 w1233 w1240 w1243] -> w46
      tunnel: w44 -> [_ w399 _ _ _ _ _ _ _ _ _ _ _ _ _ _ _ _ _ _ _ _ _ _ _ _ _ _ _ _]
      frame "Main", Default {
        n15 = event shown="[21] \"Cancel Cal\": Value Change" {
          selector: _ -> [_ _ _ _ _ _ _ _ _ _ _ _ _ _ _ _ _ _ _ _ _ _ _ _]
          dyn-events: _ -> [_ _ _ _ _ _ _ _ _ _ _ _ _ _ _ _ _ _ _ _ _ _ _ _]
          timeout: 10 -> [_ _ _ _ _ _ _ _ _ _ _ _ _ _ _ _ _ _ _ _ _ _ _ _]
          tunnel: w57 -> [w68 w100 w126 w136 w154 w169 w173 _ _ _ _ _ _ w232 w257 _ w300 _ w319 w352 w358 w381 w389 w395]
          tunnel: [w66 w96 w129 w141 w148 w167 w171 w186 w194 w202 w210 w218 w221 w235 w259 w294 w298 w307 w320 w353 w356 w374 w391 w396] -> w55
          tunnel: w56 -> [w66 w97 w124 w141 w149 w167 w171 w186 w194 w202 w210 w218 w221 w237 w259 w294 w299 w308 w320 w353 w356 w374 w391 w397]
          tunnel: [w61 w101 w125 w135 w155 w168 w173 w183 w191 w199 w207 w215 string[] ["Stop Verification"] w233 w257 string[] ["Save Cal"] w300 string[] ["Calc Dev", "Cal Review"] w319 w351 w357 w381 w390 w395] -> w54
          event Timeout {
            n16 = event-data() -> ()  [unwired: 1 in, 2 out]
            n17 = Unbundle By Name(w66) -> ("debug"=w65:bool)
            n18 = case shown="False" w65 {
              tunnel: [w81 string[] []] -> w67
              tunnel: w66 -> [w78 _]
              frame False {
                n19 = Unbundle By Name(w78) -> ("Calling VI Ref"=w80:refnum<vi>)
                n20 = property class="VI"(reference=w80) -> (error out=w77:errorcluster, "Exec.State"=w79:T13)  [unwired: 1 in, 1 out]
                n21 = call <vilib>:"Clear Errors.vi"("error in (no error)"=w77) -> ()  [unwired: 5 in, 2 out]
                n22 = case shown="\"Run top level\", \"Running\"" w79 {
                  tunnel: [string[] ["Exit"] string[] []] -> w81
                  frame Default {
                  }
                  frame "Run top level", "Running" {
                  }
                }
              }
              frame True {
              }
            }
            n23 = local read "Lost Connection"() -> (w60:bool)
            n24 = local read "RIO Found"() -> (w63:bool)
            n25 = Insert Into Array(array=w68, index=0, new element=w67) -> (w62:string[])
            n26 = And(x=w63, y=w60) -> (x .and. y?=w59:bool)
            n27 = case shown="True" w59 {
              tunnel: w62 -> [w73 w76]
              tunnel: [w70 w76] -> w61
              frame True {
                # "Lost connection."
                n28 = stacked-sequence {
                  tunnel: "Lost connection to network system.\n\nCal is now terminated." ("message") -> [w74 _]
                  frame #0 {
                    n29 = One Button Dialog(message=w74) -> ()  [unwired: 1 in, 1 out]
                  }
                  frame #1 {
                    n30 = Wait (ms)(milliseconds to wait=u32 500) -> ()  [unwired: 1 out]
                  }
                }
                n31 = Insert Into Array(array=w73, index=0, new element=string[] ["End Cal"]) -> (w70:string[])
              }
              frame False {
                # "Or not yet connected"
                # "Still connected."
              }
            }
          }
          event "Start Cal": Value Change {
            w92 = T10."Disabled and Grayed Out" ("Disabled")
            n32 = event-data() -> ()  [unwired: 1 in, 1 out]
            n33 = Unbundle By Name(w97) -> ("Registered Systems"=w89:T3[], "DAQ Rack"=w88:string)
            n34 = property on="Start Cal" class="Bool"("DisabledEnum"=w92) -> (error out=w91:errorcluster)  [unwired: 2 in, 1 out]
            n35 = property on="Header" class="Bool"("DisabledEnum"=w92) -> ()  [unwired: 2 in, 2 out]
            n36 = for {
              tunnel: w89 -> [w103] mode=indexing
              tunnel: w88 -> [w106]
              tunnel: [w104] -> w87
              tunnel: [w103] -> w86
              stop <- w105 stop-if-true
              n37 = Unbundle By Name(w103) -> ("Serial Number"=w104:u32, "ID"=w107:string)
              n38 = Equal?(x=w107, y=w106) -> (x = y?=w105:bool)
            }
            n39 = property class="DAQmx System"(error in=w91) -> (error out=w94:errorcluster, "DevNames"=w99:tag[])  [unwired: 1 in, 1 out]
            n40 = case shown="No Error" w94 {
              tunnel: w87 -> [w108 _]
              tunnel: w99 -> [w112 _]
              tunnel: [w111 -1 ("index of element")] -> w98
              tunnel: [w110 tag ""] -> w95
              frame No Error {
                n41 = for {
                  tunnel: w112 -> [w115] mode=indexing
                  tunnel: [w114] -> w109 mode=indexing
                  n42 = property class="DAQmx Device"("Active Device"=w115) -> (error out=w113:errorcluster, "DevSerialNum"=w114:u32)  [unwired: 2 in, 1 out]
                  n43 = call <vilib>:"Clear Errors.vi"("error in (no error)"=w113) -> ()  [unwired: 5 in, 2 out]
                }
                n44 = Search 1D Array(1D array=w109, element=w108) -> (index of element=w111:i32)  [unwired: 1 in]
                n45 = Index Array(array=w112, index=w111) -> (element=w110:tag)
              }
              frame Error {
              }
            }
            n46 = case shown="-1" w98 {
              tunnel: [string[] ["Load Targets", "Start Cal"] string[] ["Check for RIO", "Load Targets", "Start Cal"]] -> w102
              tunnel: "Start Cal" -> [_ _]
              frame 0, Default {
              }
              frame -1 {
              }
            }
            n47 = Bundle By Name(cluster=w97, "Verification"=FALSE, "Selected Chassis"=w95, "Desired System"=w86) -> (w96:T9)
            n48 = Insert Into Array(array=w100, index=0, new element=w102) -> (w101:string[])
          }
          event Value Change {
            n49 = event-data() -> ()  [unwired: 1 in, 6 out]
            n50 = Unbundle By Name(w124) -> ("Cal Target Array"=w123:string[])
            n51 = Index Array(array=w123, index="Channel to Cal") -> (element=w122:string)
            n52 = case shown="\"A\"" w122 {
              tunnel: [Units_Type_Def_(DAQ_Rack)."V" ("Cal Unit") Units_Type_Def_(DAQ_Rack)."A" ("Cal Unit")] -> w120
              frame "V", Default {
              }
              frame "A" {
              }
            }
            n53 = local write "Cal Unit"(w120) -> ()
            n54 = Bundle By Name(cluster=w124, "Channel to Cal"="Channel to Cal", "Cal Unit"=w120) -> (w129:T9)
            n55 = Insert Into Array(array=w126, index=0, new element=string[] ["Adjust Channels", "Load Targets"]) -> (w125:string[])
          }
          event "Header": Value Change {
            w139 = string[][] [] ("Header Table 1")
            w138 = TRUE ("Visible")
            n56 = event-data() -> ()  [unwired: 1 in, 6 out]
            n57 = property on="Main Tab" class="TabCtl (strict)"("DisabledEnum"=T10."Disabled and Grayed Out" ("Disabled")) -> ()  [unwired: 2 in, 2 out]
            n58 = property on="Header Tab" class="TabCtl (strict)"("Visible"=w138) -> ()  [unwired: 2 in, 2 out]
            n59 = property on="Load Indicator Tab" class="TabCtl (strict)"("Visible"=w138) -> ()  [unwired: 2 in, 2 out]
            n60 = local write "Tank IP:"("" ("DAQ Rack")) -> ()
            n61 = local write "RIO Found"(FALSE ("RIO Found")) -> ()
            n62 = local write "Header Table 1"(w139) -> ()
            n63 = local write "Header Table 2"(w139) -> ()
            n64 = local write "Sys Cal Table"(w139) -> ()
            n65 = local write "Cal Standards Table"(w139) -> ()
            n66 = local write "Header Comments"(w139) -> ()
            n67 = Insert Into Array(array=w136, index=0, new element=string[] ["Init Cal"]) -> (w135:string[])
          }
          event "Header OK": Value Change {
            w142 = New_Channel_Type_Def_(RIO)."AI-00/08 Pos 1 Pump Voltage" ("Channel to Cal 2")
            w147 = Units_Type_Def_(DAQ_Rack)."A" ("Cal Unit")
            w158 = T10."Disabled and Grayed Out" ("Disabled")
            n68 = event-data() -> ()  [unwired: 1 in, 1 out]
            n69 = local read "Header Table 1"() -> (w152:string[][])
            n70 = Index Array(array=w152, index (row)=3, index (col)=0 ("disabled index (col)")) -> (element=w144:string)
            "Tank IP:" <- w144
            n71 = Decimal String To Number(string=w144) -> (number=w143:i32)  [unwired: 2 in, 1 out]
            n72 = String Length(string=w144) -> (length=w146:i32)
            n73 = case shown="3" w146 {
              tunnel: [w161 System_Type."RIO" ("Desired System.System Type")] -> w145
              tunnel: w143 -> [w162 _]
              frame 4, Default {
                n74 = case shown="1000..1999" w162 {
                  tunnel: [System_Type."DAQ Rack" ("Desired System.System Type") System_Type."DAQ Cart" ("Desired System.System Type")] -> w161
                  frame Default {
                  }
                  frame 1000..1999 {
                  }
                }
              }
              frame 3 {
              }
            }
            n75 = property on="Header OK" class="Bool"("DisabledEnum"=w158) -> ()  [unwired: 2 in, 2 out]
            n76 = property on="Header Cancel" class="Bool"("DisabledEnum"=w158) -> ()  [unwired: 2 in, 2 out]
            n77 = property on="Load Indicator Tab" class="TabCtl (strict)"("Visible"=TRUE) -> ()  [unwired: 2 in, 2 out]
            n78 = disable-structure shown="Enabled" {
              disable-tunnel: [string[] ["Adjust Channels", "Create Spreadsheet", "Create Cal File", "Check for RIO"] string[] ["Adjust Channels", "Create Spreadsheet", "Create Cal File"]] -> w156
              frame Disabled {
              }
              frame Enabled {
              }
            }
            n79 = Bundle By Name(cluster=w149, "Desired System.System Type"=w145, "Desired System.ID"=w144, "DAQ Rack"=w144, "Channel to Cal"=w142, "Cal Unit"=w147) -> (w148:T9)
            n80 = local write "Channel to Cal"(w142) -> ()
            n81 = local write "Cal Unit"(w147) -> ()
            n82 = Insert Into Array(array=w154, index=0, new element=w156) -> (w155:string[])
          }
          event "Header Cancel": Value Change {
            n83 = event-data() -> ()  [unwired: 1 in, 1 out]
            n84 = Insert Into Array(array=w169, index=0, new element=string[] ["End Cal"]) -> (w168:string[])
          }
          event "View Spreadsheet": Value Change {
            n85 = event-data() -> ()  [unwired: 1 in, 1 out]
            n86 = Unbundle By Name(w171) -> ("Cal Spreadsheet Path"=w172:path)
            n87 = flat-sequence {
              tunnel: w172 -> [w176]
              frame #0 {
                n88 = property on="Main Tab" class="TabCtl (strict)"("DisabledEnum"=T10."Disabled" ("Disabled")) -> ()  [unwired: 2 in, 2 out]
                n89 = property on="Load Indicator Tab" class="TabCtl (strict)"("Visible"=TRUE) -> ()  [unwired: 2 in, 2 out]
              }
              frame #1 {
                n90 = call "Open Office File.vi"("Selection a Word (.doc, .docx), Excel (.xls, .xlsx), or Powerpoint (.ppt, .pptx) Document..."=w176) -> ()  [unwired: 10 in, 1 out]
              }
              frame #2 {
                n91 = property on="Load Indicator Tab" class="TabCtl (strict)"("Visible"=FALSE) -> ()  [unwired: 2 in, 2 out]
                n92 = property on="Main Tab" class="TabCtl (strict)"("DisabledEnum"=T10."Enabled" ("Disabled")) -> ()  [unwired: 2 in, 2 out]
              }
            }
          }
          event "1st Point Cal": Value Change {
            n93 = event-data() -> ()  [unwired: 1 in, 1 out]
            n94 = Select(t=T10."Disabled" ("Disabled"), s="1st Point Cal", f=T10."Enabled" ("Disabled")) -> (s? t:f=w182:T10)
            n95 = property on="Cal Value 1" class="DigNum (strict)"("DisabledEnum"=w182) -> ()  [unwired: 2 in, 2 out]
            n96 = property on="Cal Value 2" class="DigNum (strict)"("DisabledEnum"=w182) -> ()  [unwired: 2 in, 2 out]
            n97 = property on="Cal Value 3" class="DigNum (strict)"("DisabledEnum"=w182) -> ()  [unwired: 2 in, 2 out]
            n98 = property on="Cal Value 4" class="DigNum (strict)"("DisabledEnum"=w182) -> ()  [unwired: 2 in, 2 out]
            n99 = property on="Cal Value 5" class="DigNum (strict)"("DisabledEnum"=w182) -> ()  [unwired: 2 in, 2 out]
            n100 = property on="2nd Point Cal" class="Bool (strict)"("DisabledEnum"=w182) -> ()  [unwired: 2 in, 2 out]
            n101 = property on="3rd Point Cal" class="Bool (strict)"("DisabledEnum"=w182) -> ()  [unwired: 2 in, 2 out]
            n102 = property on="4th Point Cal" class="Bool (strict)"("DisabledEnum"=w182) -> ()  [unwired: 2 in, 2 out]
            n103 = property on="5th Point Cal" class="Bool (strict)"("DisabledEnum"=w182) -> ()  [unwired: 2 in, 2 out]
            n104 = Select(t=string[] ["Calibrating 1"], s="1st Point Cal", f=string[] ["Stop Calibrating"]) -> (s? t:f=w183:string[])
          }
          event "2nd Point Cal": Value Change {
            n105 = event-data() -> ()  [unwired: 1 in, 1 out]
            n106 = Select(t=T10."Disabled" ("Disabled"), s="2nd Point Cal", f=T10."Enabled" ("Disabled")) -> (s? t:f=w190:T10)
            n107 = property on="Cal Value 1" class="DigNum (strict)"("DisabledEnum"=w190) -> ()  [unwired: 2 in, 2 out]
            n108 = property on="Cal Value 2" class="DigNum (strict)"("DisabledEnum"=w190) -> ()  [unwired: 2 in, 2 out]
            n109 = property on="Cal Value 3" class="DigNum (strict)"("DisabledEnum"=w190) -> ()  [unwired: 2 in, 2 out]
            n110 = property on="Cal Value 4" class="DigNum (strict)"("DisabledEnum"=w190) -> ()  [unwired: 2 in, 2 out]
            n111 = property on="Cal Value 5" class="DigNum (strict)"("DisabledEnum"=w190) -> ()  [unwired: 2 in, 2 out]
            n112 = property on="1st Point Cal" class="Bool (strict)"("DisabledEnum"=w190) -> ()  [unwired: 2 in, 2 out]
            n113 = property on="3rd Point Cal" class="Bool (strict)"("DisabledEnum"=w190) -> ()  [unwired: 2 in, 2 out]
            n114 = property on="4th Point Cal" class="Bool (strict)"("DisabledEnum"=w190) -> ()  [unwired: 2 in, 2 out]
            n115 = property on="5th Point Cal" class="Bool (strict)"("DisabledEnum"=w190) -> ()  [unwired: 2 in, 2 out]
            n116 = Select(t=string[] ["Calibrating 2"], s="2nd Point Cal", f=string[] ["Stop Calibrating"]) -> (s? t:f=w191:string[])
          }
          event "3rd Point Cal": Value Change {
            n117 = event-data() -> ()  [unwired: 1 in, 1 out]
            n118 = Select(t=T10."Disabled" ("Disabled"), s="3rd Point Cal", f=T10."Enabled" ("Disabled")) -> (s? t:f=w198:T10)
            n119 = property on="Cal Value 1" class="DigNum (strict)"("DisabledEnum"=w198) -> ()  [unwired: 2 in, 2 out]
            n120 = property on="Cal Value 2" class="DigNum (strict)"("DisabledEnum"=w198) -> ()  [unwired: 2 in, 2 out]
            n121 = property on="Cal Value 3" class="DigNum (strict)"("DisabledEnum"=w198) -> ()  [unwired: 2 in, 2 out]
            n122 = property on="Cal Value 4" class="DigNum (strict)"("DisabledEnum"=w198) -> ()  [unwired: 2 in, 2 out]
            n123 = property on="Cal Value 5" class="DigNum (strict)"("DisabledEnum"=w198) -> ()  [unwired: 2 in, 2 out]
            n124 = property on="1st Point Cal" class="Bool (strict)"("DisabledEnum"=w198) -> ()  [unwired: 2 in, 2 out]
            n125 = property on="2nd Point Cal" class="Bool (strict)"("DisabledEnum"=w198) -> ()  [unwired: 2 in, 2 out]
            n126 = property on="4th Point Cal" class="Bool (strict)"("DisabledEnum"=w198) -> ()  [unwired: 2 in, 2 out]
            n127 = property on="5th Point Cal" class="Bool (strict)"("DisabledEnum"=w198) -> ()  [unwired: 2 in, 2 out]
            n128 = Select(t=string[] ["Calibrating 3"], s="3rd Point Cal", f=string[] ["Stop Calibrating"]) -> (s? t:f=w199:string[])
          }
          event "4th Point Cal": Value Change {
            n129 = event-data() -> ()  [unwired: 1 in, 6 out]
            n130 = Select(t=T10."Disabled" ("Disabled"), s="4th Point Cal", f=T10."Enabled" ("Disabled")) -> (s? t:f=w206:T10)
            n131 = property on="Cal Value 1" class="DigNum (strict)"("DisabledEnum"=w206) -> ()  [unwired: 2 in, 2 out]
            n132 = property on="Cal Value 2" class="DigNum (strict)"("DisabledEnum"=w206) -> ()  [unwired: 2 in, 2 out]
            n133 = property on="Cal Value 3" class="DigNum (strict)"("DisabledEnum"=w206) -> ()  [unwired: 2 in, 2 out]
            n134 = property on="Cal Value 4" class="DigNum (strict)"("DisabledEnum"=w206) -> ()  [unwired: 2 in, 2 out]
            n135 = property on="Cal Value 5" class="DigNum (strict)"("DisabledEnum"=w206) -> ()  [unwired: 2 in, 2 out]
            n136 = property on="1st Point Cal" class="Bool (strict)"("DisabledEnum"=w206) -> ()  [unwired: 2 in, 2 out]
            n137 = property on="2nd Point Cal" class="Bool (strict)"("DisabledEnum"=w206) -> ()  [unwired: 2 in, 2 out]
            n138 = property on="3rd Point Cal" class="Bool (strict)"("DisabledEnum"=w206) -> ()  [unwired: 2 in, 2 out]
            n139 = property on="5th Point Cal" class="Bool (strict)"("DisabledEnum"=w206) -> ()  [unwired: 2 in, 2 out]
            n140 = Select(t=string[] ["Calibrating 4"], s="4th Point Cal", f=string[] ["Stop Calibrating"]) -> (s? t:f=w207:string[])
          }
          event "5th Point Cal": Value Change {
            n141 = event-data() -> ()  [unwired: 1 in, 6 out]
            n142 = Select(t=T10."Disabled" ("Disabled"), s="5th Point Cal", f=T10."Enabled" ("Disabled")) -> (s? t:f=w214:T10)
            n143 = property on="Cal Value 1" class="DigNum (strict)"("DisabledEnum"=w214) -> ()  [unwired: 2 in, 2 out]
            n144 = property on="Cal Value 2" class="DigNum (strict)"("DisabledEnum"=w214) -> ()  [unwired: 2 in, 2 out]
            n145 = property on="Cal Value 3" class="DigNum (strict)"("DisabledEnum"=w214) -> ()  [unwired: 2 in, 2 out]
            n146 = property on="Cal Value 4" class="DigNum (strict)"("DisabledEnum"=w214) -> ()  [unwired: 2 in, 2 out]
            n147 = property on="Cal Value 5" class="DigNum (strict)"("DisabledEnum"=w214) -> ()  [unwired: 2 in, 2 out]
            n148 = property on="1st Point Cal" class="Bool (strict)"("DisabledEnum"=w214) -> ()  [unwired: 2 in, 2 out]
            n149 = property on="2nd Point Cal" class="Bool (strict)"("DisabledEnum"=w214) -> ()  [unwired: 2 in, 2 out]
            n150 = property on="3rd Point Cal" class="Bool (strict)"("DisabledEnum"=w214) -> ()  [unwired: 2 in, 2 out]
            n151 = property on="4th Point Cal" class="Bool (strict)"("DisabledEnum"=w214) -> ()  [unwired: 2 in, 2 out]
            n152 = Select(t=string[] ["Calibrating 5"], s="5th Point Cal", f=string[] ["Stop Calibrating"]) -> (s? t:f=w215:string[])
          }
          event "Cancel Verify": Value Change {
            n153 = event-data() -> ()  [unwired: 1 in, 1 out]
            n154 = Unbundle By Name(w221) -> ("StreamCtrlActive"=w219:bool, "Desired System.ID"=w220:string)
            n155 = case shown="True" w219 {
              tunnel: w220 -> [_ w223]
              frame False {
              }
              frame True {
                w224 = FALSE
                n156 = Format Into String(format string="ni.var.psp://10.30.189.%s/Streaming Control/StreamCalibrated", w223) -> (resulting string=w230:string, error out=w231:errorcluster)  [unwired: 2 in]
                n157 = shared-variable-open(w230, w231, w224) -> (w225:refnum<k21>, w228:errorcluster)  [unwired: 1 in]
                n158 = shared-variable-write(w225, w228, w224) -> (w226:refnum<k21>, w227:errorcluster)
                n159 = Close Variable Connection(8:w227, 11:w226) -> ()  [unwired: 1 out]
              }
            }
          }
          event "Verify Read": Value Change {
            n160 = event-data() -> ()  [unwired: 1 in, 1 out]
            n161 = case shown="False" "Verify Read" {
              tunnel: [FALSE ("Verify Read") FALSE ("Verify Read")] -> w238
              tunnel: w237 -> [_ _]
              tunnel: w237 -> [w242 w248]
              tunnel: [w242 w247] -> w236
              tunnel: [w240 string[] ["Calc Dev", "Cal Review"]] -> w233
              tunnel: w232 -> [w240 _]
              frame False {
              }
              frame True {
                n162 = local read "Ver Reading"() -> (w243:dbl)
                n163 = local read "Verify Table"() -> (w244:string[][])
                n164 = local read "Row"() -> (w251:i32)
                n165 = Number To Fractional String(number=w243) -> (F-format string=w250:string)  [unwired: 3 in]
                n166 = Replace Array Subset(array=w244, new element=w250, index (row)=w251, index (col)=1 ("disabled index (col)")) -> (w246:string[][])
                n167 = Increment(x=w251) -> (x+1=w255:i32)
                n168 = Bundle(w255, "disabled index (col)"=1) -> (w252:cluster{i32, "disabled index (col)":i32})  [unwired: 1 in]
                n169 = Bundle By Name(cluster=w248, "Verify Table"=w246) -> (w247:T9)
                n170 = property on="Verify Table" class="Tbl (strict)"("Key Focus"=TRUE, "EditPos"=w252, "Value"=w246) -> ()  [unwired: 2 in, 2 out]
              }
            }
            n171 = local write "Verify Read"(w238) -> ()
            n172 = Bundle By Name(cluster=w236, "Init Mean"=TRUE ("initialize")) -> (w235:T9)
          }
          event "Verify Edit": Value Change {
            n173 = event-data() -> ()  [unwired: 1 in, 1 out]
            n174 = case shown="False" "Verify Edit" {
              tunnel: w259 -> [w272 _]
              frame False {
                w273 = T10."Enabled" ("Disabled")
                n175 = Unbundle By Name(w272) -> ("Targets"=w268:T6, "Cal Targets Path"=w270:path, "Cal Unit"=w269:T2)
                n176 = local read "Verify Table"() -> (w271:string[][])
                n177 = Index Array(array=w271, index (col)=0 ("disabled index (col)")) -> (element=w262:string[])  [unwired: 1 in]
                n178 = Fract/Exp String To Number(string=w262) -> (number=w261:dbl[])  [unwired: 3 in, 1 out]
                n179 = Array To Cluster(array=w261) -> (cluster=w260:T14)
                n180 = case shown="\"A\"" w269 {
                  tunnel: w268 -> [w278 w281 w284 w287 w290]
                  tunnel: [w277 w280 w283 w286 w289] -> w267
                  tunnel: w260 -> [w276 w279 w282 w285 w288]
                  frame "V", Default {
                    n181 = Bundle By Name(cluster=w278, "V Targets"=w276) -> (w277:T6)
                  }
                  frame "mA" {
                    n182 = Bundle By Name(cluster=w281, "mA Targets"=w279) -> (w280:T6)
                  }
                  frame "A" {
                    n183 = Bundle By Name(cluster=w284, "A Targets"=w282) -> (w283:T6)
                  }
                  frame "Hz" {
                    n184 = Bundle By Name(cluster=w287, "Hz Targets"=w285) -> (w286:T6)
                  }
                  frame "deg C" {
                    n185 = Bundle By Name(cluster=w290, "TC Targets"=w288) -> (w289:T6)
                  }
                }
                n186 = call <vilib>:"Open Config Data.vi"("configuration file path"=w270) -> ("error out"=w266:errorcluster, "refnum"=w265:T15)  [unwired: 8 in, 1 out]
                n187 = call <userlib>:"Write INI Cluster__ogtk.vi"("error in (no error)"=w266, "INI Fomatted Cluster"=w267, "refnum"=w265) -> ("error out"=w264:errorcluster, "dup refnum"=w263:T15)  [unwired: 7 in]
                n188 = property on="Hide Cal Values" class="Bool"("Visible"=TRUE) -> ()  [unwired: 2 in, 2 out]
                n189 = call <vilib>:"Close Config Data.vi"("error in (no error)"=w264, "refnum"=w263) -> ()  [unwired: 8 in, 2 out]
                n190 = property on="Verify Read" class="Bool (strict)"("DisabledEnum"=w273) -> ()  [unwired: 2 in, 2 out]
                n191 = property on="Auto" class="Bool (strict)"("DisabledEnum"=w273) -> ()  [unwired: 2 in, 2 out]
              }
              frame True {
                w291 = T10."Disabled and Grayed Out" ("Disabled")
                n192 = property on="Verify Read" class="Bool (strict)"("DisabledEnum"=w291) -> ()  [unwired: 2 in, 2 out]
                n193 = property on="Auto" class="Bool (strict)"("DisabledEnum"=w291) -> ()  [unwired: 2 in, 2 out]
                n194 = property on="Hide Cal Values" class="Bool"("Visible"=FALSE) -> ()  [unwired: 2 in, 2 out]
              }
            }
          }
          event "Save Cal": Value Change {
            n195 = event-data() -> ()  [unwired: 1 in, 1 out]
            n196 = property on="Cal Table" class="Tbl (strict)"("DisabledEnum"=T10."Enabled" ("Disabled")) -> ()  [unwired: 2 in, 2 out]
            n197 = property on="Verify Tab" class="TabCtl (strict)"("Visible"=FALSE) -> ()  [unwired: 2 in, 2 out]
          }
          event "Auto": Value Change {
            n198 = event-data() -> ()  [unwired: 1 in, 1 out]
            n199 = case shown="True" "Auto" {
              frame False {
              }
              frame True {
                n200 = local read "Row"() -> (w301:i32)
                n201 = Bundle("Row"=w301, "disabled index (col)"=1) -> (w302:cluster{"Row":i32, "disabled index (col)":i32})  [unwired: 1 in]
                n202 = property on="Verify Table" class="Tbl (strict)"("Key Focus"=TRUE, "EditPos"=w302) -> ()  [unwired: 2 in, 2 out]
              }
            }
            n203 = Bundle By Name(cluster=w299, "Auto"="Auto") -> (w298:T9)
          }
          event "Verify Table": Value Change {
            n204 = event-data() -> ()  [unwired: 1 in, 1 out]
            n205 = Bundle By Name(cluster=w308, "Verify Table"="Verify Table") -> (w307:T9)
          }
          event "Confirm Cal Point": Value Change {
            w313 = T10."Enabled" ("Disabled")
            n206 = event-data() -> ()  [unwired: 1 in, 1 out]
            n207 = local read "Cal Reading"() -> (w317:dbl)
            n208 = Unbundle By Name(w320) -> ("LastCalPt"=w318:i32)
            n209 = flat-sequence {
              tunnel: w318 -> [w324]
              tunnel: w317 -> [w323]
              tunnel: FALSE -> [w322]
              tunnel: "Master Value" -> [w321]
              tunnel: [w340] -> w312
              frame #0 {
                n210 = case shown="0, Default" w324 {
                  tunnel: w323 -> [_ w325 w328 w331 w334 w337]
                  tunnel: w321 -> [_ w327 w330 w333 w336 w339]
                  tunnel: w322 -> [_ w326 w329 w332 w335 w338]
                  frame 0, Default {
                  }
                  frame 1 {
                    n211 = local write "Cal Value 1"(w327) -> ()
                    n212 = local write "1st Point Cal"(w326) -> ()
                    "Reading Value 1" <- w325
                  }
                  frame 2 {
                    n213 = local write "Cal Value 2"(w330) -> ()
                    n214 = local write "2nd Point Cal"(w329) -> ()
                    "Reading Value 2" <- w328
                  }
                  frame 3 {
                    n215 = local write "Cal Value 3"(w333) -> ()
                    n216 = local write "3rd Point Cal"(w332) -> ()
                    "Reading Value 3" <- w331
                  }
                  frame 4 {
                    n217 = local write "Cal Value 4"(w336) -> ()
                    n218 = local write "4th Point Cal"(w335) -> ()
                    "Reading Value 4" <- w334
                  }
                  frame 5 {
                    n219 = local write "Cal Value 5"(w339) -> ()
                    n220 = local write "5th Point Cal"(w338) -> ()
                    "Reading Value 5" <- w337
                  }
                }
              }
              frame #1 {
                n221 = local read "Reading Value 2"() -> (w345:dbl)
                n222 = local read "Reading Value 3"() -> (w346:dbl)
                n223 = local read "Reading Value 4"() -> (w347:dbl)
                n224 = local read "Reading Value 5"() -> (w348:dbl)
                n225 = Not Equal To 0?(x=w345) -> (x != 0?=w344:bool)
                n226 = Not Equal To 0?(x=w346) -> (x != 0?=w343:bool)
                n227 = Not Equal To 0?(x=w347) -> (x != 0?=w342:bool)
                n228 = Not Equal To 0?(x=w348) -> (x != 0?=w341:bool)
                n229 = Compound Arithmetic op=AND(w344, w343, w342, w341) -> (w340:bool)
              }
            }
            n230 = property on="Cal Value 1" class="DigNum (strict)"("DisabledEnum"=w313) -> ()  [unwired: 2 in, 2 out]
            n231 = property on="Cal Value 2" class="DigNum (strict)"("DisabledEnum"=w313) -> ()  [unwired: 2 in, 2 out]
            n232 = property on="Cal Value 3" class="DigNum (strict)"("DisabledEnum"=w313) -> ()  [unwired: 2 in, 2 out]
            n233 = property on="Cal Value 4" class="DigNum (strict)"("DisabledEnum"=w313) -> ()  [unwired: 2 in, 2 out]
            n234 = property on="Cal Value 5" class="DigNum (strict)"("DisabledEnum"=w313) -> ()  [unwired: 2 in, 2 out]
            n235 = property on="1st Point Cal" class="Bool (strict)"("DisabledEnum"=w313) -> ()  [unwired: 2 in, 2 out]
            n236 = property on="2nd Point Cal" class="Bool (strict)"("DisabledEnum"=w313) -> ()  [unwired: 2 in, 2 out]
            n237 = property on="3rd Point Cal" class="Bool (strict)"("DisabledEnum"=w313) -> ()  [unwired: 2 in, 2 out]
            n238 = property on="4th Point Cal" class="Bool (strict)"("DisabledEnum"=w313) -> ()  [unwired: 2 in, 2 out]
            n239 = property on="5th Point Cal" class="Bool (strict)"("DisabledEnum"=w313) -> ()  [unwired: 2 in, 2 out]
            n240 = local write "Cal Tab"(enum32{"Apply", "Cal"}."Apply" ("Cal Tab")) -> ()
            n241 = Select(t=T10."Enabled" ("Disabled"), s=w312, f=T10."Disabled and Grayed Out" ("Disabled")) -> (s? t:f=w309:T10)
            n242 = property on="Apply Cal" class="Bool"("DisabledEnum"=w309) -> ()  [unwired: 2 in, 2 out]
          }
          event "Apply Cal": Value Change {
            n243 = event-data() -> ()  [unwired: 1 in, 6 out]
            n244 = Insert Into Array(array=w352, index=0, new element=string[] ["Calculate Coeffs"]) -> (w351:string[])
          }
          event "Start Verification": Value Change {
            n245 = event-data() -> ()  [unwired: 1 in, 6 out]
            n246 = Unbundle By Name(w356) -> ("StreamCtrlActive"=w354:bool, "Desired System.ID"=w355:string)
            n247 = case shown="True" w354 {
              tunnel: w355 -> [_ w362]
              frame False {
              }
              frame True {
                n248 = Format Into String(format string="ni.var.psp://10.30.189.%s/Streaming Control/StreamCalibrated", w362) -> (resulting string=w370:string, error out=w371:errorcluster)  [unwired: 2 in]
                n249 = shared-variable-open(w370, w371, FALSE) -> (w364:refnum<k21>, w367:errorcluster)  [unwired: 1 in]
                n250 = shared-variable-write(w364, w367, TRUE ("data in")) -> (w365:refnum<k21>, w366:errorcluster)
                n251 = Close Variable Connection(8:w366, 11:w365) -> ()  [unwired: 1 out]
              }
            }
            n252 = property on="Verify Tab" class="TabCtl (strict)"("Visible"="Start Verification") -> ()  [unwired: 2 in, 2 out]
            n253 = Insert Into Array(array=w358, index=0, new element=string[] ["Load Targets", "Calculate Coeffs"]) -> (w357:string[])
          }
          event "Cancel Cal": Value Change {
            w382 = T10."Disabled and Grayed Out" ("Disabled")
            w383 = T10."Enabled" ("Disabled")
            n254 = event-data() -> ()  [unwired: 1 in, 6 out]
            n255 = Unbundle By Name(w374) -> ("Desired System.ID"=w377:string)
            n256 = Format Into String(format string="10.30.189.%s", w377) -> (resulting string=w373:string)  [unwired: 2 in, 1 out]
            n257 = flat-sequence {
              tunnel: w373 -> [w385]
              tunnel: [w385] -> w375
              tunnel: [w388] -> w372
              tunnel: w375 -> [w388]
              frame #0 {
                n258 = local write "RIO Found"(FALSE ("RIO Found")) -> ()
              }
              frame #1 {
                n259 = Wait (ms)(milliseconds to wait=u32 20) -> ()  [unwired: 1 out]
              }
            }
            n260 = property on="Cal Tab" class="TabCtl (strict)"("Visible"=FALSE) -> ()  [unwired: 2 in, 2 out]
            n261 = property on="Cal Unit" class="Enum (strict)"("DisabledEnum"=T10."Enabled" ("Disabled")) -> ()  [unwired: 2 in, 2 out]
            n262 = property on="Header" class="Bool"("DisabledEnum"=w383) -> ()  [unwired: 2 in, 2 out]
            n263 = property on="Channel to Cal" class="Enum (strict)"("DisabledEnum"=w383) -> ()  [unwired: 2 in, 2 out]
            n264 = property on="View Spreadsheet" class="Bool"("DisabledEnum"=w383) -> ()  [unwired: 2 in, 2 out]
            n265 = property on="Start Cal" class="Bool"("DisabledEnum"=w383) -> ()  [unwired: 2 in, 2 out]
            n266 = call "TCP Data Stream PC.vi"("RT IP Address"=w372, "Mode"=TCP_Data_Stream_Mode_(PC)."Close") -> ()  [unwired: 14 in, 4 out]
            n267 = disable-structure shown="Disabled" {
              disable-tunnel: w383 -> [w384 _]
              frame Disabled {
                n268 = property on="Start Verification" class="Bool"("DisabledEnum"=w384) -> ()  [unwired: 2 in, 2 out]
              }
              frame Enabled {
              }
            }
            n269 = property on="Reading Value 1" class="DigNum (strict)"("DisabledEnum"=w382) -> ()  [unwired: 2 in, 2 out]
            n270 = property on="Cal Value 1" class="DigNum (strict)"("DisabledEnum"=w382) -> ()  [unwired: 2 in, 2 out]
            n271 = property on="1st Point Cal" class="Bool (strict)"("DisabledEnum"=w382) -> ()  [unwired: 2 in, 2 out]
            n272 = property on="Reading Value 2" class="DigNum (strict)"("DisabledEnum"=w382) -> ()  [unwired: 2 in, 2 out]
            n273 = property on="Cal Value 2" class="DigNum (strict)"("DisabledEnum"=w382) -> ()  [unwired: 2 in, 2 out]
            n274 = property on="2nd Point Cal" class="Bool (strict)"("DisabledEnum"=w382) -> ()  [unwired: 2 in, 2 out]
            n275 = property on="Reading Value 3" class="DigNum (strict)"("DisabledEnum"=w382) -> ()  [unwired: 2 in, 2 out]
            n276 = property on="Cal Value 3" class="DigNum (strict)"("DisabledEnum"=w382) -> ()  [unwired: 2 in, 2 out]
            n277 = property on="3rd Point Cal" class="Bool (strict)"("DisabledEnum"=w382) -> ()  [unwired: 2 in, 2 out]
            n278 = property on="Reading Value 4" class="DigNum (strict)"("DisabledEnum"=w382) -> ()  [unwired: 2 in, 2 out]
            n279 = property on="Cal Value 4" class="DigNum (strict)"("DisabledEnum"=w382) -> ()  [unwired: 2 in, 2 out]
            n280 = property on="4th Point Cal" class="Bool (strict)"("DisabledEnum"=w382) -> ()  [unwired: 2 in, 2 out]
            n281 = property on="Reading Value 5" class="DigNum (strict)"("DisabledEnum"=w382) -> ()  [unwired: 2 in, 2 out]
            n282 = property on="Cal Value 5" class="DigNum (strict)"("DisabledEnum"=w382) -> ()  [unwired: 2 in, 2 out]
            n283 = property on="5th Point Cal" class="Bool (strict)"("DisabledEnum"=w382) -> ()  [unwired: 2 in, 2 out]
          }
          event "Transfer Cal": Value Change {
            n284 = event-data() -> ()  [unwired: 1 in, 6 out]
            n285 = disable-structure shown="Disabled" {
              disable-tunnel: [string[] ["Distribute Calibration"] w393] -> w390
              disable-tunnel: w389 -> [_ w393]
              frame Disabled {
              }
              frame Enabled {
              }
            }
          }
          event Value Change {
            n286 = event-data() -> ()  [unwired: 1 in, 1 out]
            n287 = Bundle By Name(cluster=w397, "Cal Unit"="Cal Unit") -> (w396:T9)
          }
        }
      }
      frame "Init" {
        w402 = FALSE ("Visible")
        w409 = Units_Type_Def_(DAQ_Rack)."A" ("Cal Unit")
        # "#Change adding in\nnew subVI for RIO"
        n288 = Unbundle By Name(w418) -> ("debug"=w417:bool, "App Dir"=w416:path)
        n289 = Select(t=path "C:/Users/zstreeter/Documents/Projects/Calibration Utility/Source", s=w417, f=w416) -> (s? t:f=w415:path)
        n290 = Build Path(base path=w415, name or relative path="App Config.ini") -> (appended path=w421:path)
        n291 = Build Path(base path=w415, name or relative path="Calibration UIs\\New Durability Tank") -> (appended path=w413:path)
        n292 = call "Read App Config.vi"("App Config Path"=w421) -> ("Cal Files Path"=w424:path, "Registered Systems"=w411:T3[])  [unwired: 9 in]
        n293 = Build Path(base path=w424, name or relative path="New Durability Tank") -> (appended path=w420:path)
        n294 = Build Path(base path=w413, name or relative path="New Cal Targets.ini") -> (appended path=w423:path)
        n295 = Create Folder(path (use dialog)=w420) -> (error out=w426:errorcluster)  [unwired: 2 in, 2 out]
        n296 = call <vilib>:"Clear Errors.vi"("error in (no error)"=w426) -> ("error out"=w419:errorcluster)  [unwired: 5 in, 1 out]
        n297 = for {
          tunnel: [w434] -> w412 mode=indexing
          tunnel: w420 -> [w433]
          tunnel: w419 -> [w432]
          tunnel: w413 -> [w431]
          tunnel: string[] ["New Durability Tank Cal Template.xls"] -> [w430] mode=indexing
          n298 = Build Path(base path=w433, name or relative path=w430) -> (appended path=w434:path)
          n299 = Build Path(base path=w431, name or relative path=w430) -> (appended path=w437:path)
          n300 = call <vilib>:"Check if File or Folder Exists.vi"("error in (no error)"=w432, "path"=w434) -> ("file or folder exists?"=w435:bool, "dup path"=w436:path)  [unwired: 7 in, 1 out]
          n301 = case shown="True" w435 {
            tunnel: w436 -> [w439 _]
            tunnel: w437 -> [w438 _]
            frame False {
              n302 = Copy(10:w439, 11:w438) -> ()  [unwired: 3 in, 3 out]
            }
            frame True {
            }
          }
        }
        n303 = Index Array(array=w412) -> (element=w408:path)  [unwired: 1 in]
        n304 = call "New Create Cal File Array (RIO).vi"() -> ("Cal Target Array"=w404:string[], "Cal Log OUT"=w403:string[][])  [unwired: 10 in]
        n305 = Bundle By Name(cluster=w418, "Registered Systems"=w411, "Cal Files Base Path"=w420, "Base Path"=w415, "Cal Targets Path"=w423, "Cal Template Path"=w408, "Default Cal Log"=w403, "Cal Target Array"=w404, "Cal Unit"=w409) -> (w401:T9)
        n306 = property on="Cal Tab" class="TabCtl (strict)"("Visible"=w402) -> ()  [unwired: 2 in, 2 out]
        n307 = property on="Verify Tab" class="TabCtl (strict)"("Visible"=w402) -> ()  [unwired: 2 in, 2 out]
        n308 = local write "Tank IP:"("" ("DAQ Rack")) -> ()
        n309 = local write "Cal Table"(string[][] []) -> ()
        n310 = local write "Cal Unit"(w409) -> ()
        n311 = flat-sequence {
          tunnel: w401 -> [w429]
          tunnel: [w429] -> w400
          tunnel: w399 -> [w428]
          frame #0 {
            n312 = Set Occurrence(w428) -> ()
          }
        }
      }
      frame "Unused Items" {
      }
      frame "Init Cal" {
        w444 = FALSE ("Auto")
        w450 = FALSE ("Verify Read")
        w451 = T10."Enabled" ("Disabled")
        w443 = FALSE ("Visible")
        w442 = T10."Disabled and Grayed Out" ("Disabled")
        n313 = Unbundle By Name(w454) -> ("Cal Log Header"=w446:string[])
        n314 = property on="Cal Table" class="Tbl (strict)"("Column Headers[]"=w446) -> ()  [unwired: 2 in, 2 out]
        n315 = property on="Reading Value 1" class="DigNum (strict)"("DisabledEnum"=w442) -> ()  [unwired: 2 in, 2 out]
        n316 = property on="Cal Value 1" class="DigNum (strict)"("DisabledEnum"=w442) -> ()  [unwired: 2 in, 2 out]
        n317 = property on="1st Point Cal" class="Bool (strict)"("DisabledEnum"=w442) -> ()  [unwired: 2 in, 2 out]
        n318 = property on="Reading Value 2" class="DigNum (strict)"("DisabledEnum"=w442) -> ()  [unwired: 2 in, 2 out]
        n319 = property on="Cal Value 2" class="DigNum (strict)"("DisabledEnum"=w442) -> ()  [unwired: 2 in, 2 out]
        n320 = property on="2nd Point Cal" class="Bool (strict)"("DisabledEnum"=w442) -> ()  [unwired: 2 in, 2 out]
        n321 = property on="Reading Value 3" class="DigNum (strict)"("DisabledEnum"=w442) -> ()  [unwired: 2 in, 2 out]
        n322 = property on="Cal Value 3" class="DigNum (strict)"("DisabledEnum"=w442) -> ()  [unwired: 2 in, 2 out]
        n323 = property on="3rd Point Cal" class="Bool (strict)"("DisabledEnum"=w442) -> ()  [unwired: 2 in, 2 out]
        n324 = property on="Reading Value 4" class="DigNum (strict)"("DisabledEnum"=w442) -> ()  [unwired: 2 in, 2 out]
        n325 = property on="Cal Value 4" class="DigNum (strict)"("DisabledEnum"=w442) -> ()  [unwired: 2 in, 2 out]
        n326 = property on="4th Point Cal" class="Bool (strict)"("DisabledEnum"=w442) -> ()  [unwired: 2 in, 2 out]
        n327 = property on="Reading Value 5" class="DigNum (strict)"("DisabledEnum"=w442) -> ()  [unwired: 2 in, 2 out]
        n328 = property on="Cal Value 5" class="DigNum (strict)"("DisabledEnum"=w442) -> ()  [unwired: 2 in, 2 out]
        n329 = property on="5th Point Cal" class="Bool (strict)"("DisabledEnum"=w442) -> ()  [unwired: 2 in, 2 out]
        n330 = property on="Verify Read" class="Bool (strict)"("DisabledEnum"=w451) -> ()  [unwired: 2 in, 2 out]
        n331 = property on="Cal Table" class="Tbl (strict)"("DisabledEnum"=w451) -> ()  [unwired: 2 in, 2 out]
        n332 = property on="Verify Tab" class="TabCtl (strict)"("Visible"=w443) -> ()  [unwired: 2 in, 2 out]
        n333 = property on="Cal Tab" class="TabCtl (strict)"("Visible"=w443) -> ()  [unwired: 2 in, 2 out]
        n334 = property on="Hide Cal Values" class="Bool"("Visible"=TRUE) -> ()  [unwired: 2 in, 2 out]
        n335 = local write "Verify Read"(w450) -> ()
        n336 = local write "Auto"(w450) -> ()
        n337 = local write "Verify Edit"(w450) -> ()
        n338 = Bundle By Name(cluster=w454, "Auto"=w444, "Verification"=w444) -> (w453:T9)
        n339 = Insert Into Array(array=w448, index=0, new element=string[] ["Clear Dev Data", "Update Dev Tables", "Load Template"]) -> (w445:string[])
      }
      frame "Check for RIO" {
        n340 = Unbundle By Name(w461) -> ("Desired System.Serial Number"=w455:u32, "Desired System.ID"=w457:string, "Verification"=w459:bool, "StreamCtrlActive"=w458:bool)
        n341 = local read "RIO Found"() -> (w456:bool)
        n342 = case shown="False" w456 {
          selector: w456 -> [w467 _]
          tunnel: [string[] [] w475] -> w462
          tunnel: [w467 w474] -> w460
          tunnel: w459 -> [_ w473]
          tunnel: w458 -> [_ w472]
          tunnel: w457 -> [_ w471]
          tunnel: w455 -> [_ w468]
          frame True {
          }
          frame False {
            n343 = call "Find Network Systems.vi"() -> ("Serial Number"=w470:u32)  [unwired: 10 in, 1 out]
            n344 = Equal?(x=w470, y=w468) -> (x = y?=w469:bool)
            n345 = case shown="True" w469 {
              selector: w469 -> [w478 w494]
              tunnel: w473 -> [w479 _]
              tunnel: [w480 string[] []] -> w475
              tunnel: [w478 w494] -> w474
              tunnel: w471 -> [w477 _]
              tunnel: w472 -> [w476 _]
              frame True {
                # "Desired system found."
                n346 = case shown="True" w476 {
                  tunnel: w477 -> [_ w481]
                  frame False {
                  }
                  frame True {
                    w482 = FALSE
                    n347 = Format Into String(format string="ni.var.psp://10.30.189.%s/Streaming Control/StreamCalibrated", w481) -> (resulting string=w488:string, error out=w489:errorcluster)  [unwired: 2 in]
                    n348 = shared-variable-open(w488, w489, w482) -> (w483:refnum<k21>, w486:errorcluster)  [unwired: 1 in]
                    n349 = shared-variable-write(w483, w486, w482) -> (w484:refnum<k21>, w485:errorcluster)
                    n350 = Close Variable Connection(8:w485, 11:w484) -> ()  [unwired: 1 out]
                  }
                }
                n351 = case shown="False" w479 {
                  tunnel: [string[] ["Load Targets", "Calculate Coeffs"] w491] -> w480
                  frame True {
                  }
                  frame False {
                    n352 = disable-structure shown="Enabled" {
                      disable-tunnel: [string[] ["Load Targets", "Start Cal"] string[] ["Load Targets"]] -> w491
                      frame Disabled {
                      }
                      frame Enabled {
                      }
                    }
                  }
                }
              }
              frame False {
                # "Couldn't find desired system."
                n353 = property on="Header" class="Bool"("DisabledEnum"=T10."Enabled" ("Disabled")) -> ()  [unwired: 2 in, 2 out]
                n354 = One Button Dialog(message="Couldn't connect to desired DAQ hardware.") -> ()  [unwired: 1 in, 1 out]
              }
            }
          }
        }
        "RIO Found" <- w460
        n355 = Insert Into Array(array=w464, index=0, new element=w462) -> (w463:string[])
      }
      frame "Adjust Channels" {
        n356 = Unbundle By Name(w512) -> ("Cal Unit"=w506:T2)
        n357 = property on="Channel to Cal" class="Enum (strict)"() -> ("NumItems"=w504:u32)  [unwired: 2 in, 2 out]
        n358 = property on="Cal Unit" class="Enum (strict)"() -> ("Strings []"=w509:string[])  [unwired: 2 in, 2 out]
        n359 = for {
          N: w504 -> [_]
          shift-right: [w526] -> w501
          shift-left: i32[] [] ("Disabled Items []") -> [w527]
          i -> [w525]
          n360 = case shown="54..63" w525 {
            tunnel: w527 -> [w528 w531]
            tunnel: [w528 w529] -> w526
            tunnel: w525 -> [_ w530]
            frame 0..53, Default {
            }
            frame 54..63 {
              n361 = Build Array (concatenate)(w531, w530) -> (w529:i32[])
            }
          }
        }
        n362 = for {
          tunnel: w509 -> [w520] mode=indexing
          shift-right: [w518] -> w500
          shift-left: i32[] [] ("Disabled Items []") -> [w519]
          i -> [w517]
          n363 = case shown="\"Hz\", \"deg C\", \"mA\"" w520 {
            tunnel: w519 -> [w521 w524]
            tunnel: [w521 w522] -> w518
            tunnel: w517 -> [_ w523]
            frame "A", "V", Default {
            }
            frame "Hz", "deg C", "mA" {
              n364 = Build Array (concatenate)(w524, w523) -> (w522:i32[])
            }
          }
        }
        n365 = Search 1D Array(1D array=w500, element=w506) -> (index of element=w508:i32)  [unwired: 1 in]
        n366 = disable-structure shown="Enabled" {
          disable-tunnel: w501 -> [w515 _]
          disable-tunnel: w500 -> [w514 _]
          disable-tunnel: [w515 w516] -> w499
          disable-tunnel: [w514 w516] -> w498
          frame Disabled {
          }
          frame Enabled {
            w516 = i32[] [] ("Disabled Items []")
          }
        }
        n367 = Greater Or Equal To 0?(x=w508) -> (x >= 0?=w507:bool)
        n368 = case shown="True" w507 {
          tunnel: [w532 w533] -> w505
          tunnel: w506 -> [w532 _]
          tunnel: w500 -> [_ w535]
          frame False {
          }
          frame True {
            n369 = for {
              N: 5 -> [_]
              tunnel: w535 -> [w539]
              tunnel: [w536] -> w533
              i -> [w536]
              stop <- w537 stop-if-true
              n370 = Search 1D Array(1D array=w539, element=w536) -> (index of element=w538:i32)  [unwired: 1 in]
              n371 = Less Than 0?(x=w538) -> (x < 0?=w537:bool)
            }
            n372 = local write "Cal Unit"(w533) -> ()
          }
        }
        n373 = property on="Channel to Cal" class="Enum (strict)"("Disabled Items []"=w499) -> ()  [unwired: 2 in, 2 out]
        n374 = property on="Cal Unit" class="Enum (strict)"("Disabled Items []"=w498) -> ()  [unwired: 2 in, 2 out]
        n375 = Bundle By Name(cluster=w512, "Rack Version"=Rack_Version_Type_Def."RIO", "Cal Unit"=w505) -> (w511:T9)
      }
      frame "Clear Dev Data" {
        n376 = Bundle By Name(cluster=w542, "Verify Table"=string[][] [["", "", "", "", ""], ["", "", "", "", ""], ["", "", "", "", ""], ["", "", "", "", ""], ["", "", "", "", ""], ["", "", "", "", ""], ["", "", "", "", ""], ["", "", "", "", ""], ["", "", "", "", ""], ["", "", "", "", ""]]) -> (w541:T9)
      }
      frame "Update Dev Tables" {
        n377 = Unbundle By Name(w545) -> ("Verify Table"=w544:string[][])
        n378 = local write "Verify Table"(w544) -> ()
      }
      frame "Load Template" {
        n379 = Unbundle By Name(w548) -> ("Cal Template Path"=w553:path)
        n380 = call <vilib>:"Check if File or Folder Exists.vi"("path"=w553) -> ("file or folder exists?"=w552:bool)  [unwired: 8 in, 2 out]
        n381 = case shown="False" w552 {
          tunnel: [string[] [] string[] []] -> w551
          tunnel: w553 -> [w560 w563]
          tunnel: [FALSE ("Visible") FALSE ("Visible")] -> w554
          tunnel: [w557 w565] -> w555
          tunnel: [w557 w565] -> w556
          frame False {
            w557 = T10."Disabled and Grayed Out" ("Disabled")
            n382 = Format Into String(format string="Can't find cal spreadsheet template!\n\nShould have been here:  \"%s\"" ("message"), w560) -> (resulting string=w559:string)  [unwired: 2 in, 1 out]
            n383 = One Button Dialog(message=w559) -> ()  [unwired: 1 in, 1 out]
          }
          frame True {
            w565 = T10."Enabled" ("Disabled")
            n384 = call "Read Write Header.vi"("Cal Template Path"=w563, "Write (F)"=FALSE) -> ("Header Table 1"=w571:string[][], "Header Table 2"=w570:string[][], "Sys Cal Table"=w567:string[][], "Cal Standards Table"=w566:string[][], "Header Comments"=w568:string[][])  [unwired: 13 in]
            n385 = local write "Header Table 1"(w571) -> ()
            n386 = local write "Header Table 2"(w570) -> ()
            n387 = local write "Sys Cal Table"(w567) -> ()
            n388 = local write "Cal Standards Table"(w566) -> ()
            n389 = local write "Header Comments"(w568) -> ()
          }
        }
        n390 = property on="Load Indicator Tab" class="TabCtl (strict)"("Visible"=w554) -> ()  [unwired: 2 in, 2 out]
        n391 = property on="Header OK" class="Bool"("DisabledEnum"=w555) -> ()  [unwired: 2 in, 2 out]
        n392 = property on="Header Cancel" class="Bool"("DisabledEnum"=w556) -> ()  [unwired: 2 in, 2 out]
        n393 = Insert Into Array(array=w550, index=0, new element=w551) -> (w549:string[])
      }
      frame "Create Spreadsheet" {
        n394 = Unbundle By Name(w584) -> ("Rack Version"=w579:T5, "DAQ Rack"=w576:string, "Cal Files Base Path"=w586:path)
        n395 = Format Into String(format string="%s.xls", w576) -> (resulting string=w575:string)  [unwired: 2 in, 1 out]
        n396 = case shown="\"RIO\"" w579 {
          tunnel: ["DAQ Rack Cal Template.xls" ("name or relative path") "DAQ Cart Cal Template.xls" ("name or relative path") "New Durability Tank Cal Template.xls" ("name or relative path")] -> w574
          frame Default {
          }
          frame "Cart" {
          }
          frame "RIO" {
          }
        }
        n397 = Build Path(base path=w586, name or relative path=w575) -> (appended path=w573:path)
        n398 = Empty String/Path?(string/path=w576) -> (empty?=w578:bool)
        n399 = Not A Number/Path/Refnum?(number/path/refnum=w573) -> (NaN/Path/Refnum?=w588:bool)
        n400 = Or(x=w588, y=w578) -> (x .or. y?=w589:bool)
        n401 = Build Path(base path=w586, name or relative path=w574) -> (appended path=w587:path)
        n402 = case shown="True" w589 {
          tunnel: [string[] ["Save Header"] string[] []] -> w585
          tunnel: w573 -> [w594 _]
          tunnel: w587 -> [w595 _]
          frame False {
            n403 = call <vilib>:"Check if File or Folder Exists.vi"("path"=w594) -> ("file or folder exists?"=w593:bool)  [unwired: 8 in, 2 out]
            n404 = case shown="False" w593 {
              tunnel: w594 -> [w599 _]
              tunnel: w595 -> [w598 _]
              frame False {
                n405 = Copy(9:TRUE ("overwrite (F)"), 10:w599, 11:w598) -> ()  [unwired: 2 in, 3 out]
              }
              frame True {
              }
            }
          }
          frame True {
            w600 = T10."Enabled" ("Disabled")
            n406 = property on="Load Indicator Tab" class="TabCtl (strict)"("Visible"=FALSE) -> ()  [unwired: 2 in, 2 out]
            n407 = property on="Header OK" class="Bool"("DisabledEnum"=w600) -> ()  [unwired: 2 in, 2 out]
            n408 = property on="Header Cancel" class="Bool"("DisabledEnum"=w600) -> ()  [unwired: 2 in, 2 out]
            n409 = One Button Dialog(message="\"Manufacturer Serial #\" is blank or contains invalid characters.") -> ()  [unwired: 1 in, 1 out]
          }
        }
        n410 = Bundle By Name(cluster=w584, "Cal Spreadsheet Path"=w573) -> (w583:T9)
        n411 = Insert Into Array(array=w581, index=0, new element=w585) -> (w582:string[])
      }
      frame "Save Header" {
        n412 = Unbundle By Name(w612) -> ("Cal Spreadsheet Path"=w615:path, "Cal Template Path"=w616:path)
        n413 = Build Array(w615, w616) -> (w617:path[])
        n414 = for {
          tunnel: "Header Table 2" -> [w625]
          tunnel: "Sys Cal Table" -> [w624]
          tunnel: "Cal Standards Table" -> [w623]
          tunnel: "Header Comments" -> [w622]
          tunnel: [w621] -> w614
          tunnel: "Header Table 1" -> [w619]
          tunnel: w617 -> [w618] mode=indexing
          n415 = call "Read Write Header.vi"("Header Table 1 IN"=w619, "Header Table 2 IN"=w625, "Sys Cal Table IN"=w624, "Cal Standards Table IN"=w623, "Header Comments IN"=w622, "Cal Template Path"=w618, "Write (F)"=TRUE) -> ("Header Table 1"=w621:string[][])  [unwired: 8 in, 4 out]
        }
        n416 = flat-sequence {
          tunnel: w614 -> [_]
          frame #0 {
            w627 = T10."Enabled" ("Disabled")
            w628 = FALSE ("Visible")
            n417 = disable-structure shown="Disabled" {
              disable-tunnel: w627 -> [w629 _]
              frame Disabled {
                n418 = property on="Start Verification" class="Bool"("DisabledEnum"=w629) -> ()  [unwired: 2 in, 2 out]
              }
              frame Enabled {
              }
            }
            n419 = property on="View Spreadsheet" class="Bool"("DisabledEnum"=w627) -> ()  [unwired: 2 in, 2 out]
            n420 = property on="Main Tab" class="TabCtl (strict)"("DisabledEnum"=w627) -> ()  [unwired: 2 in, 2 out]
            n421 = property on="Tank IP:" class="Str"("DisabledEnum"=w627) -> ()  [unwired: 2 in, 2 out]
            n422 = property on="Channel to Cal" class="Enum (strict)"("DisabledEnum"=w627) -> ()  [unwired: 2 in, 2 out]
            n423 = property on="Start Cal" class="Bool"("DisabledEnum"=w627) -> ()  [unwired: 2 in, 2 out]
            n424 = property on="Cal Unit" class="Enum (strict)"("DisabledEnum"=T10."Enabled" ("Disabled")) -> ()  [unwired: 2 in, 2 out]
            n425 = property on="Load Indicator Tab" class="TabCtl (strict)"("Visible"=w628) -> ()  [unwired: 2 in, 2 out]
            n426 = property on="Header Tab" class="TabCtl (strict)"("Visible"=w628) -> ()  [unwired: 2 in, 2 out]
          }
        }
        n427 = Insert Into Array(array=w610, index=0, new element=string[] []) -> (w611:string[])
      }
      frame "Create Cal File" {
        n428 = Unbundle By Name(w633) -> ("Cal Files Base Path"=w635:path, "Cal Log Header"=w638:string[], "Default Cal Log"=w637:string[][])
        n429 = local read "Tank IP:"() -> (w630:string)
        n430 = Build Array (concatenate)(w638, w637) -> (w636:string[][])
        n431 = case shown="Default" w630 {
          tunnel: w636 -> [w647 _]
          tunnel: w635 -> [w646 _]
          tunnel: w630 -> [w644 _]
          tunnel: [w645 path "" ("dup path")] -> w631
          frame Default {
            n432 = Format Into String(format string="%s.cal", w644) -> (resulting string=w642:string)  [unwired: 2 in, 1 out]
            n433 = Build Path(base path=w646, name or relative path=w642) -> (appended path=w650:path)
            n434 = call <vilib>:"Check if File or Folder Exists.vi"("path"=w650) -> ("file or folder exists?"=w649:bool, "dup path"=w648:path)  [unwired: 8 in, 1 out]
            n435 = case shown="False" w649 {
              tunnel: w648 -> [w654 w655]
              tunnel: w647 -> [w653 _]
              tunnel: [w651 w655] -> w645
              frame False {
                n436 = call-poly <vilib>:"Write To Spreadsheet File.vi"("delimiter (\\t)"="," ("delimiter (\\t)"), "2D data"=w653, "file path (dialog if empty)"=w654) -> ("new file path (Not A Path if cancelled)"=w651:path)  [unwired: 5 in]
              }
              frame True {
              }
            }
          }
          frame "" {
          }
        }
        n437 = Bundle By Name(cluster=w633, "Cal File Path"=w631) -> (w632:T9)
        n438 = Insert Into Array(array=w639, index=0, new element=string[] ["Load Cal File"]) -> (w640:string[])
      }
      frame "Load Cal File" {
        n439 = Unbundle By Name(w661) -> ("Default Cal Log"=w657:string[][], "Cal File Path"=w658:path)
        n440 = Empty String/Path?(string/path=w658) -> (empty?=w659:bool)
        n441 = case shown="False" w659 {
          tunnel: w658 -> [w668 _]
          tunnel: [w672 w709] -> w665
          tunnel: [w670 string[] []] -> w662
          tunnel: w661 -> [w669 w709]
          tunnel: w657 -> [w666 _]
          frame False {
            n442 = call <vilib>:"Check if File or Folder Exists.vi"("path"=w668) -> ("file or folder exists?"=w671:bool, "dup path"=w667:path)  [unwired: 8 in, 1 out]
            n443 = case shown="True" w671 {
              tunnel: w667 -> [_ w703]
              tunnel: w669 -> [w673 w700]
              tunnel: [w673 w699] -> w672
              tunnel: [string[] ["Create Cal File"] string[] []] -> w670
              tunnel: w666 -> [_ w696]
              frame False {
              }
              frame True {
                w695 = 0 ("index (row)")
                n444 = call-poly <vilib>:"Read From Spreadsheet File.vi"("delimiter (\\t)"="," ("delimiter (\\t)"), "file path (dialog if empty)"=w703) -> ("all rows"=w702:string[][])  [unwired: 5 in, 4 out]
                n445 = Delete From Array(array=w702, index (row)=0) -> (array with subset deleted=w691:string[][])  [unwired: 2 in, 1 out]
                n446 = Index Array(array=w691, index (col)=0 ("disabled index (col)")) -> (element=w693:string[])  [unwired: 1 in]
                n447 = Search 1D Array(1D array=w693, element="") -> (index of element=w689:i32)  [unwired: 1 in]
                n448 = Delete From Array(array=w691, index (row)=w689) -> (array with subset deleted=w690:string[][])  [unwired: 2 in, 1 out]
                n449 = Replace Array Subset(array=w696, new element=w690, index (row)=w695, index (col)=w695) -> (w683:string[][])
                n450 = Index Array(array=w683, index (col)=1 ("disabled index (col)")) -> (element=w676:string[])  [unwired: 1 in]
                n451 = for {
                  tunnel: w676 -> [w705] mode=indexing
                  tunnel: [w704] -> w675 mode=indexing
                  n452 = case shown="\"V\", Default" w705 {
                    tunnel: ["V" "A"] -> w704
                    frame "V", Default {
                    }
                    frame "A" {
                    }
                  }
                }
                n453 = Array To Spreadsheet String(array=w675, 3:"%s" ("format string")) -> (spreadsheet string=w687:string)  [unwired: 1 in]
                n454 = Search and Replace String(replace all?=TRUE ("replace all? (F)"), input string=w687, search string="degC", replace string="deg C" ("search string")) -> (result string=w680:string)  [unwired: 4 in, 3 out]
                n455 = Spreadsheet String To Array(format string="%s", spreadsheet string=w680, array type (2D Dbl)=w675) -> (array=w679:string[])  [unwired: 1 in]
                n456 = Replace Array Subset(array=w683, new element=w679, index (col)=1 ("disabled index (col)")) -> (w682:string[][])  [unwired: 1 in]
                n457 = Bundle By Name(cluster=w700, "Cal Log"=w682) -> (w699:T9)
                n458 = property on="Cal Table" class="Tbl (strict)"("Value"=w682) -> ()  [unwired: 2 in, 2 out]
              }
            }
          }
          frame True {
          }
        }
        n459 = Insert Into Array(array=w663, index=0, new element=w662) -> (w664:string[])
      }
      frame "Load Targets" {
        w766 = 0 ("length")
        # "#Change In \"A\" selection added selection of \"RIO\" that links 25A Targets and Setpoints"
        n460 = Unbundle By Name(w769) -> ("Cal Log"=w734:string[][], "Cal Targets Path"=w776:path, "Targets"=w771:T6, "Cal Target Array"=w756:string[], "Verify Table"=w723:string[][], "Channel to Cal"=w745:T1)
        n461 = property on="Cancel Verify" class="Bool"("DisabledEnum"=T10."Enabled" ("Disabled")) -> ()  [unwired: 2 in, 2 out]
        n462 = property on="Cal Table" class="Tbl (strict)"("Active Cell"=T12 {"Row"=-2, "Column"=-2} ("Active Cell:Active Cell"), "Cell BG Color"=u32 16448250) -> ()  [unwired: 2 in, 2 out]
        n463 = Index Array(array=w734, index (row)=w745) -> (element=w755:string[])  [unwired: 1 in]
        n464 = call <vilib>:"Open Config Data.vi"("configuration file path"=w776) -> ("error out"=w774:errorcluster, "refnum"=w775:T15)  [unwired: 8 in, 1 out]
        n465 = Array Subset "Calibration"(array=w755, index=2, length=10) -> (w718:string[])
        n466 = Array Subset "Verification"(array=w755, index=18, length=20) -> (w725:string[])
        n467 = property on="Apply Cal" class="Bool"("DisabledEnum"=T10."Disabled and Grayed Out" ("Disabled")) -> ()  [unwired: 2 in, 2 out]
        n468 = call <userlib>:"Read INI Cluster__ogtk.vi"("error in (no error)"=w774, "INI Fomatted Cluster Type"=w771, "refnum"=w775) -> ("error out"=w772:errorcluster, "INI Fomatted Cluster"=w770:variant, "dup refnum"=w773:T15)  [unwired: 4 in, 2 out]
        n469 = Index Array(array=w725, index #1=1 ("index"), index #2=3 ("index"), index #3=5 ("index"), index #4=7 ("index"), index #5=9 ("index")) -> (element #1=w744:string, element #2=w741:string, element #3=w743:string, element #4=w740:string, element #5=w742:string)
        n470 = call <vilib>:"Close Config Data.vi"("error in (no error)"=w772, "refnum"=w773) -> ()  [unwired: 8 in, 2 out]
        n471 = Fract/Exp String To Number(string=w718) -> (number=w728:dbl[])  [unwired: 3 in, 1 out]
        n472 = Empty Array?(array=w718) -> ()  [unwired: 1 out]
        n473 = Empty String/Path?(string/path=w744) -> (empty?=w737:bool)
        n474 = Empty String/Path?(string/path=w743) -> (empty?=w736:bool)
        n475 = Empty String/Path?(string/path=w742) -> (empty?=w735:bool)
        n476 = Variant To Data(type=w771, Variant=w770) -> (data=w759:T6)  [unwired: 1 in, 1 out]
        n477 = Index Array(array=w756, index=w745) -> (element=w760:string)
        n478 = Empty String/Path?(string/path=w741) -> (empty?=w739:bool)
        n479 = Empty String/Path?(string/path=w740) -> (empty?=w738:bool)
        n480 = Compound Arithmetic op=AND(w737, w739, w736, w738, w735) -> (w719:bool)
        n481 = case shown="\"DegC\"" w760 {
          tunnel: w759 -> [w824 w827 w830 w833 w836 w839]
          tunnel: [w822 w825 w828 w831 w834 w837] -> w757
          tunnel: [w823 w826 w829 w832 w835 w838] -> w758
          frame "V", Default {
            n482 = Unbundle By Name(w824) -> ("V Targets"=w823:T7, "V Setpoints"=w822:T8)
          }
          frame "A" {
            n483 = Unbundle By Name(w827) -> ("A Targets"=w826:T7, "A Setpoints"=w825:T8)
          }
          frame "DegC" {
            n484 = Unbundle By Name(w830) -> ("DegC Targets"=w829:T7, "DegC Setpoints"=w828:T8)
          }
          frame "kPa" {
            n485 = Unbundle By Name(w833) -> ("kPa Targets"=w832:T7, "kPa Setpoints"=w831:T8)
          }
          frame "LpH" {
            n486 = Unbundle By Name(w836) -> ("LpH Targets"=w835:T7, "LpH Setpoints"=w834:T8)
          }
          frame "CT" {
            n487 = Unbundle By Name(w839) -> ("CT Targets"=w838:T7, "CT Setpoints"=w837:T8)
          }
        }
        n488 = case shown="True" w719 {
          tunnel: w725 -> [_ w797]
          tunnel: w723 -> [w789 w796]
          tunnel: [w789 w790] -> w722
          frame True {
          }
          frame False {
            n489 = for {
              tunnel: w797 -> [w803] mode=indexing
              tunnel: [w803] -> w792 mode=indexing if=w799
              tunnel: [w803] -> w791 mode=indexing if=w798
              i -> [w802]
              n490 = Quotient & Remainder(x=w802, y=2) -> (x-y*floor(x/y)=w800:i32)  [unwired: 1 out]
              n491 = Equal To 0?(x=w800) -> (x = 0?=w799:bool)
              n492 = Not(x=w799) -> (.not. x?=w798:bool)
            }
            n493 = Replace Array Subset(array=w796, new element=w792, index (col)=0 ("disabled index (col)")) -> (w795:string[][])  [unwired: 1 in]
            n494 = Replace Array Subset(array=w795, new element=w791, index (col)=1 ("disabled index (col)")) -> (w790:string[][])  [unwired: 1 in]
          }
        }
        n495 = case shown="False" w719 {
          tunnel: w721 -> [w786 w788]
          tunnel: [w785 w788] -> w720
          frame False {
            n496 = Insert Into Array(array=w786, index=0, new element=string[] ["Calc Dev"]) -> (w785:string[])
          }
          frame True {
          }
        }
        n497 = for {
          tunnel: w718 -> [w783] mode=indexing
          tunnel: [w782] -> w717 mode=indexing
          n498 = Empty String/Path?(string/path=w783) -> (empty?=w782:bool)
        }
        n499 = Cluster To Array(cluster=w758) -> (array=w767:dbl[])
        n500 = Cluster To Array(cluster=w757) -> (array=w724:dbl[])
        n501 = And Array Elements(Boolean array=w717) -> (logical AND=w716:bool)
        n502 = Delete From Array(array=w767, length=w766, index=w766) -> (deleted portion=w762:dbl[], array with subset deleted=w765:dbl[])
        n503 = call-poly <userlib>:"Remove Duplicates from 1D Array__ogtk.vi"("Input Array"=w765) -> ("Output Array"=w764:dbl[])  [unwired: 1 out]
        n504 = Build Array (concatenate)(w762, w764) -> (w763:dbl[])
        n505 = Number To Fractional String(number=w763, precision (6)=i16 3) -> (F-format string=w768:string[])  [unwired: 2 in]
        n506 = case shown="False" w716 {
          tunnel: w724 -> [_ w821]
          tunnel: [w809 w820] -> w733
          tunnel: [w813 w819] -> w732
          tunnel: [w812 w818] -> w731
          tunnel: [w811 w817] -> w730
          tunnel: [w810 w816] -> w729
          tunnel: w728 -> [w814 _]
          tunnel: [w808 w815] -> w715
          tunnel: [w807 w815] -> w714
          tunnel: [w806 w815] -> w713
          tunnel: [w805 w815] -> w712
          tunnel: [w804 w815] -> w711
          frame False {
            n507 = Index Array(array=w814) -> (element #1=w808:dbl, element #2=w813:dbl, element #3=w807:dbl, element #4=w812:dbl, element #5=w806:dbl, element #6=w811:dbl, element #7=w805:dbl, element #8=w810:dbl, element #9=w804:dbl, element #10=w809:dbl)  [unwired: 10 in]
          }
          frame True {
            w815 = 0.0 ("Label")
            n508 = Index Array(array=w821) -> (element #1=w819:dbl, element #2=w818:dbl, element #3=w817:dbl, element #4=w816:dbl, element #5=w820:dbl)  [unwired: 5 in]
          }
        }
        n509 = Replace Array Subset(array=w723, new element=w768, index (col)=0 ("disabled index (col)")) -> (w727:string[][])  [unwired: 1 in]
        n510 = Select(t=w727, s=w719, f=w722) -> (s? t:f=w726:string[][])
        n511 = local write "Reading Value 1"(w715) -> ()
        n512 = local write "Reading Value 2"(w714) -> ()
        n513 = local write "Reading Value 3"(w713) -> ()
        n514 = local write "Reading Value 4"(w712) -> ()
        n515 = local write "Reading Value 5"(w711) -> ()
        n516 = local write "Cal Value 1"(w732) -> ()
        n517 = local write "Cal Value 2"(w731) -> ()
        n518 = local write "Cal Value 3"(w730) -> ()
        n519 = local write "Cal Value 4"(w729) -> ()
        n520 = local write "Cal Value 5"(w733) -> ()
        n521 = Bundle By Name(cluster=w769, "Targets"=w759, "Verify Table"=w726) -> (w778:T9)
        n522 = property on="Verify Table" class="Tbl (strict)"("Value"=w726) -> ()  [unwired: 2 in, 2 out]
      }
      frame "Start Cal" {
        w842 = T10."Disabled and Grayed Out" ("Disabled")
        w843 = T10."Enabled" ("Disabled")
        n523 = property on="Header" class="Bool"("DisabledEnum"=w842) -> ()  [unwired: 2 in, 2 out]
        n524 = property on="Channel to Cal" class="Enum (strict)"("DisabledEnum"=w842) -> ()  [unwired: 2 in, 2 out]
        n525 = property on="View Spreadsheet" class="Bool"("DisabledEnum"=w842) -> ()  [unwired: 2 in, 2 out]
        n526 = property on="Cal Tab" class="TabCtl (strict)"("Visible"=TRUE) -> ()  [unwired: 2 in, 2 out]
        n527 = property on="Start Cal" class="Bool"("DisabledEnum"=w842) -> ()  [unwired: 2 in, 2 out]
        n528 = disable-structure shown="Disabled" {
          disable-tunnel: w842 -> [w845 _]
          frame Disabled {
            n529 = property on="Cal Unit" class="Enum (strict)"("DisabledEnum"=w845) -> ()  [unwired: 2 in, 2 out]
          }
          frame Enabled {
          }
        }
        n530 = property on="Start Verification" class="Bool"("DisabledEnum"=w842) -> ()  [unwired: 2 in, 2 out]
        n531 = property on="Reading Value 1" class="DigNum (strict)"("DisabledEnum"=w843) -> ()  [unwired: 2 in, 2 out]
        n532 = property on="Cal Value 1" class="DigNum (strict)"("DisabledEnum"=w843) -> ()  [unwired: 2 in, 2 out]
        n533 = property on="1st Point Cal" class="Bool (strict)"("DisabledEnum"=w843) -> ()  [unwired: 2 in, 2 out]
        n534 = property on="Reading Value 2" class="DigNum (strict)"("DisabledEnum"=w843) -> ()  [unwired: 2 in, 2 out]
        n535 = property on="Cal Value 2" class="DigNum (strict)"("DisabledEnum"=w843) -> ()  [unwired: 2 in, 2 out]
        n536 = property on="2nd Point Cal" class="Bool (strict)"("DisabledEnum"=w843) -> ()  [unwired: 2 in, 2 out]
        n537 = property on="Reading Value 3" class="DigNum (strict)"("DisabledEnum"=w843) -> ()  [unwired: 2 in, 2 out]
        n538 = property on="Cal Value 3" class="DigNum (strict)"("DisabledEnum"=w843) -> ()  [unwired: 2 in, 2 out]
        n539 = property on="3rd Point Cal" class="Bool (strict)"("DisabledEnum"=w843) -> ()  [unwired: 2 in, 2 out]
        n540 = property on="Reading Value 4" class="DigNum (strict)"("DisabledEnum"=w843) -> ()  [unwired: 2 in, 2 out]
        n541 = property on="Cal Value 4" class="DigNum (strict)"("DisabledEnum"=w843) -> ()  [unwired: 2 in, 2 out]
        n542 = property on="4th Point Cal" class="Bool (strict)"("DisabledEnum"=w843) -> ()  [unwired: 2 in, 2 out]
        n543 = property on="Reading Value 5" class="DigNum (strict)"("DisabledEnum"=w843) -> ()  [unwired: 2 in, 2 out]
        n544 = property on="Cal Value 5" class="DigNum (strict)"("DisabledEnum"=w843) -> ()  [unwired: 2 in, 2 out]
        n545 = property on="5th Point Cal" class="Bool (strict)"("DisabledEnum"=w843) -> ()  [unwired: 2 in, 2 out]
      }
      frame "Calibrating 1".."Calibrating 6" {
        # "When it said \"Calibrating 1\"..\"Calibrating 5\" it was not accepting Calibrating 5"
        n546 = case shown="\"Calibrating 4\"" w851 {
          tunnel: [0.0 w857 w859 w861 w863 w865] -> w850
          tunnel: [1 1 2 3 4 5] -> w846
          frame Default {
          }
          frame "Calibrating 1" {
            n547 = local read "Cal Value 1"() -> (w857:dbl)
          }
          frame "Calibrating 2" {
            n548 = local read "Cal Value 2"() -> (w859:dbl)
          }
          frame "Calibrating 3" {
            n549 = local read "Cal Value 3"() -> (w861:dbl)
          }
          frame "Calibrating 4" {
            n550 = local read "Cal Value 4"() -> (w863:dbl)
          }
          frame "Calibrating 5" {
            n551 = local read "Cal Value 5"() -> (w865:dbl)
          }
        }
        n552 = property on="Cal Tab" class="TabCtl (strict)"("Visible"=TRUE) -> ()  [unwired: 2 in, 2 out]
        n553 = local write "Cal Tab"(enum32{"Apply", "Cal"}."Cal" ("Cal Tab")) -> ()
        n554 = local write "Master Value"(w850) -> ()
        n555 = Bundle By Name(cluster=w848, "LastCalPt"=w846) -> (w847:T9)
      }
      frame "Stop Calibrating" {
        n556 = local write "Cal Tab"(enum32{"Apply", "Cal"}."Apply" ("Cal Tab")) -> ()
      }
      frame "Calculate Coeffs" {
        w870 = T10."Enabled" ("Disabled")
        # "Used to enable and start the verification from here"
        n557 = Unbundle By Name(w877) -> ("Channel to Cal"=w873:T1, "Cal Unit"=w876:T2, "Verification"=w875:bool, "Cal Log"=w874:string[][])
        n558 = case shown="False" w875 {
          tunnel: [w891 w918] -> w882
          tunnel: [w890 w917] -> w881
          tunnel: [w889 w916] -> w880
          tunnel: w876 -> [w888 w915]
          tunnel: w874 -> [_ w919]
          tunnel: w873 -> [_ w920]
          tunnel: [w887 w914] -> w872
          tunnel: [w886 w913] -> w871
          frame False {
            n559 = case shown="\"V\", \"Hz\", Default" w888 {
              tunnel: [w908 w911] -> w891
              tunnel: [w907 1.0] -> w890
              tunnel: [w906 w911] -> w889
              tunnel: [w901 w911] -> w887
              tunnel: [w900 w911] -> w886
              frame "V", "Hz", Default {
                n560 = local read "Reading Value 1"() -> (w899:dbl)
                n561 = local read "Reading Value 2"() -> (w898:dbl)
                n562 = local read "Reading Value 3"() -> (w897:dbl)
                n563 = local read "Reading Value 4"() -> (w895:dbl)
                n564 = local read "Reading Value 5"() -> (w894:dbl)
                n565 = Build Array("Cal Value 1", "Cal Value 2", "Cal Value 3", "Cal Value 4", "Cal Value 5") -> (w905:dbl[])
                n566 = Build Array(w899, w898, w897, w895, w894) -> (w904:dbl[])
                n567 = call <vilib>:"General Polynomial Fit Coefficients.vi"("Y"=w905, "polynomial order"=4, "X"=w904) -> ("Polynomial Coefficients"=w903:dbl[])  [unwired: 11 in, 1 out]
                n568 = Index Array(array=w903) -> (element #1=w908:dbl, element #2=w907:dbl, element #3=w906:dbl, element #4=w901:dbl, element #5=w900:dbl)  [unwired: 5 in]
              }
              frame "deg C" {
                w911 = 0.0
              }
            }
          }
          frame True {
            n569 = case shown="Default" w915 {
              selector: w915 -> [w923 _]
              tunnel: w920 -> [w939 _]
              tunnel: w919 -> [w931 _]
              tunnel: [w926 w945] -> w918
              tunnel: [w925 1.0 ("Label")] -> w917
              tunnel: [w924 w945] -> w916
              tunnel: [w922 w945] -> w914
              tunnel: [w921 w945] -> w913
              frame Default {
                n570 = Format Into String(w939) -> (resulting string=w936:string)  [unwired: 3 in, 1 out]
                n571 = Format Into String(w923) -> (resulting string=w932:string)  [unwired: 3 in, 1 out]
                n572 = Index Array(array=w931, index (col) #1=0 ("disabled index (col)"), index (col) #2=1 ("index (col)")) -> (element #1=w937:string[], element #2=w933:string[])  [unwired: 2 in]
                n573 = call-poly <userlib>:"Search Array__ogtk.vi"("Array"=w937, "Element Data"=w936) -> ("Indices of Elements"=w934:i32[])  [unwired: 7 in]
                n574 = for {
                  tunnel: w934 -> [w940] mode=indexing
                  tunnel: w933 -> [w944]
                  tunnel: w932 -> [w942]
                  tunnel: [w940] -> w930
                  stop <- w941 stop-if-true
                  n575 = Index Array(array=w944, index=w940) -> (element=w943:string)
                  n576 = Equal?(x=w942, y=w943) -> (x = y?=w941:bool)
                }
                n577 = Index Array(array=w931, index (row)=w930) -> (element=w929:string[])  [unwired: 1 in]
                n578 = Fract/Exp String To Number(string=w929) -> (number=w928:dbl[])  [unwired: 3 in, 1 out]
                n579 = Index Array(array=w928, index #1=12 ("index")) -> (element #1=w926:dbl, element #2=w925:dbl, element #3=w924:dbl, element #4=w922:dbl, element #5=w921:dbl)  [unwired: 4 in]
              }
              frame "deg C" {
                w945 = 0.0 ("Label")
              }
            }
          }
        }
        "a0" <- w882
        "a2" <- w880
        "a1" <- w881
        "a4" <- w871
        "a3" <- w872
        n580 = property on="Cal Table" class="Tbl (strict)"("DisabledEnum"=T10."Disabled and Grayed Out" ("Disabled")) -> ()  [unwired: 2 in, 2 out]
        n581 = property on="Save Cal" class="Bool"("DisabledEnum"=T10."Enabled" ("Disabled")) -> ()  [unwired: 2 in, 2 out]
        n582 = Insert Into Array(array=w883, index=0, new element=string[] ["Save Calibration"]) -> (w884:string[])
        n583 = property on="a0" class="DigNum (strict)"("DisabledEnum"=w870) -> ()  [unwired: 2 in, 2 out]
        n584 = property on="a1" class="DigNum (strict)"("DisabledEnum"=w870) -> ()  [unwired: 2 in, 2 out]
        n585 = property on="a2" class="DigNum (strict)"("DisabledEnum"=w870) -> ()  [unwired: 2 in, 2 out]
        n586 = property on="a3" class="DigNum (strict)"("DisabledEnum"=w870) -> ()  [unwired: 2 in, 2 out]
        n587 = property on="a4" class="DigNum (strict)"("DisabledEnum"=w870) -> ()  [unwired: 2 in, 2 out]
      }
      frame "Cal Review Prep" {
        w952 = T10."Disabled and Grayed Out" ("Disabled")
        n588 = Unbundle By Name(w953) -> ("Desired System.ID"=w954:string)
        n589 = Format Into String(format string="ni.var.psp://10.30.189.%s/Streaming Control/StreamCalibrated", w954) -> (resulting string=w962:string, error out=w963:errorcluster)  [unwired: 2 in]
        n590 = property on="Cal Tab" class="TabCtl (strict)"("Visible"=FALSE) -> ()  [unwired: 2 in, 2 out]
        n591 = property on="Verify Tab" class="TabCtl (strict)"("Visible"=TRUE) -> (error out=w949:errorcluster)  [unwired: 2 in, 1 out]
        n592 = shared-variable-open(w962, w963, FALSE) -> (w956:refnum<k21>, w959:errorcluster)  [unwired: 1 in]
        n593 = shared-variable-write(w956, w959, TRUE ("data in")) -> (w957:refnum<k21>, w958:errorcluster)
        n594 = property on="Verify Table" class="Tbl (strict)"(error in=w949, "Key Focus"=TRUE, "EditPos"=T12 {"Row"=0, "Column"=1} ("Active Cell:Active Cell")) -> ()  [unwired: 1 in, 2 out]
        n595 = Close Variable Connection(8:w958, 11:w957) -> ()  [unwired: 1 out]
        n596 = Insert Into Array(array=w967, index=0, new element=string[] ["Cal Review"]) -> (w966:string[])
        n597 = property on="Reading Value 1" class="DigNum (strict)"("DisabledEnum"=w952) -> ()  [unwired: 2 in, 2 out]
        n598 = property on="Cal Value 1" class="DigNum (strict)"("DisabledEnum"=w952) -> ()  [unwired: 2 in, 2 out]
        n599 = property on="1st Point Cal" class="Bool (strict)"("DisabledEnum"=w952) -> ()  [unwired: 2 in, 2 out]
        n600 = property on="Reading Value 2" class="DigNum (strict)"("DisabledEnum"=w952) -> ()  [unwired: 2 in, 2 out]
        n601 = property on="Cal Value 2" class="DigNum (strict)"("DisabledEnum"=w952) -> ()  [unwired: 2 in, 2 out]
        n602 = property on="2nd Point Cal" class="Bool (strict)"("DisabledEnum"=w952) -> ()  [unwired: 2 in, 2 out]
        n603 = property on="Reading Value 3" class="DigNum (strict)"("DisabledEnum"=w952) -> ()  [unwired: 2 in, 2 out]
        n604 = property on="Cal Value 3" class="DigNum (strict)"("DisabledEnum"=w952) -> ()  [unwired: 2 in, 2 out]
        n605 = property on="3rd Point Cal" class="Bool (strict)"("DisabledEnum"=w952) -> ()  [unwired: 2 in, 2 out]
        n606 = property on="Reading Value 4" class="DigNum (strict)"("DisabledEnum"=w952) -> ()  [unwired: 2 in, 2 out]
        n607 = property on="Cal Value 4" class="DigNum (strict)"("DisabledEnum"=w952) -> ()  [unwired: 2 in, 2 out]
        n608 = property on="4th Point Cal" class="Bool (strict)"("DisabledEnum"=w952) -> ()  [unwired: 2 in, 2 out]
        n609 = property on="Reading Value 5" class="DigNum (strict)"("DisabledEnum"=w952) -> ()  [unwired: 2 in, 2 out]
        n610 = property on="Cal Value 5" class="DigNum (strict)"("DisabledEnum"=w952) -> ()  [unwired: 2 in, 2 out]
        n611 = property on="5th Point Cal" class="Bool (strict)"("DisabledEnum"=w952) -> ()  [unwired: 2 in, 2 out]
      }
      frame "Cal Review" {
        n612 = Unbundle By Name(w978) -> ("Auto"=w976:bool, "Verify Table"=w979:string[][])
        n613 = property on="Verify Table" class="Tbl (strict)"() -> ("EditPos"=w992:T12)  [unwired: 2 in, 2 out]
        n614 = Unbundle(w992) -> ("Row"=w990:i32)  [unwired: 1 out]
        n615 = local read "Ver Reading"() -> (w969:dbl)
        n616 = Greater Or Equal To 0?(x=w990) -> (x >= 0?=w991:bool)
        n617 = Index Array(array=w979, index (row)=w990, index (col)=0 ("disabled index (col)")) -> (element=w982:string)
        n618 = Fract/Exp String To Number(string=w982) -> (number=w971:dbl)  [unwired: 3 in, 1 out]
        n619 = case shown="True" w991 {
          tunnel: w990 -> [_ w1000]
          frame False {
          }
          frame True {
            "Row" <- w1000
          }
        }
        n620 = Increment(x=w969) -> (x+1=w983:dbl)
        n621 = Increment(x=w971) -> (x+1=w984:dbl)
        n622 = Subtract(x=w983, y=w984) -> (x-y=w972:dbl)
        n623 = Divide(x=w972, y=w983) -> (x/y=w988:dbl)
        n624 = local read "Lost Connection"() -> (w968:bool)
        n625 = Empty String/Path?(string/path=w982) -> (empty?=w975:bool)
        n626 = Absolute Value(x=w988) -> (abs(x)=w970:dbl)
        n627 = Not(x=w975) -> (.not. x?=w985:bool)
        n628 = Less?(x=w970, y=0.1) -> (x < y?=w986:bool)
        n629 = Compound Arithmetic op=AND(w976, w986, w985) -> (w981:bool)
        n630 = call "Reading Delay.vi"("Delay"="ms", "In Range"=w981) -> ("Take Reading"=w974:bool)  [unwired: 9 in]
        n631 = case shown="False" w968 {
          tunnel: [string[] ["Main", "Cal Review"] string[] ["End Cal"]] -> w996
          frame False {
          }
          frame True {
          }
        }
        n632 = case shown="True" w974 {
          selector: w974 -> [_ w999]
          frame False {
          }
          frame True {
            n633 = property on="Verify Read" class="Bool (strict)"("Val(Sgnl)"=w999) -> ()  [unwired: 2 in, 2 out]
          }
        }
        n634 = Bundle By Name(cluster=w978, "Init Mean"=FALSE) -> (w973:T9)
        n635 = Insert Into Array(array=w994, index=0, new element=w996) -> (w995:string[])
      }
      frame "Stop Verification" {
        w1002 = T10."Enabled" ("Disabled")
        n636 = property on="Header" class="Bool"("DisabledEnum"=w1002) -> ()  [unwired: 2 in, 2 out]
        n637 = property on="Channel to Cal" class="Enum (strict)"("DisabledEnum"=w1002) -> ()  [unwired: 2 in, 2 out]
        n638 = property on="View Spreadsheet" class="Bool"("DisabledEnum"=w1002) -> ()  [unwired: 2 in, 2 out]
        n639 = property on="Cal Unit" class="Enum (strict)"("DisabledEnum"=T10."Enabled" ("Disabled")) -> ()  [unwired: 2 in, 2 out]
        n640 = property on="Start Cal" class="Bool"("DisabledEnum"=w1002) -> ()  [unwired: 2 in, 2 out]
        n641 = disable-structure shown="Disabled" {
          disable-tunnel: w1002 -> [w1006 _]
          frame Disabled {
            n642 = property on="Start Verification" class="Bool"("DisabledEnum"=w1006) -> ()  [unwired: 2 in, 2 out]
          }
          frame Enabled {
          }
        }
        n643 = property on="Verify Tab" class="TabCtl (strict)"("Visible"=FALSE) -> ()  [unwired: 2 in, 2 out]
      }
      frame "Save Cal" {
        w1053 = u16 4 ("y")
        n644 = Unbundle By Name(w1028) -> ("Cal File Path"=w1038:path, "Cal Log Header"=w1060:string[], "Cal Log"=w1024:string[][], "Channel to Cal"=w1036:T1, "Cal Unit"=w1037:T2, "Verification"=w1027:bool, "Verify Table"=w1039:string[][])
        n645 = local read "Reading Value 1"() -> (w1021:dbl)
        n646 = local read "Reading Value 2"() -> (w1019:dbl)
        n647 = local read "Reading Value 3"() -> (w1017:dbl)
        n648 = local read "Reading Value 4"() -> (w1015:dbl)
        n649 = local read "Reading Value 5"() -> (w1013:dbl)
        n650 = local read "Cal Value 1"() -> (w1020:dbl)
        n651 = local read "Cal Value 2"() -> (w1018:dbl)
        n652 = local read "Cal Value 3"() -> (w1016:dbl)
        n653 = local read "Cal Value 4"() -> (w1014:dbl)
        n654 = local read "Cal Value 5"() -> (w1012:dbl)
        n655 = local read "a0"() -> (w1011:dbl)
        n656 = local read "a1"() -> (w1010:dbl)
        n657 = local read "a2"() -> (w1009:dbl)
        n658 = local read "a3"() -> (w1008:dbl)
        n659 = local read "a4"() -> (w1007:dbl)
        n660 = Build Array(w1021, w1020, w1019, w1018, w1017, w1016, w1015, w1014, w1013, w1012, w1011, w1010, w1009, w1008, w1007) -> (w1066:dbl[])
        n661 = Format Into String(w1036) -> (resulting string=w1032:string)  [unwired: 3 in, 1 out]
        n662 = Format Into String(w1037) -> (resulting string=w1029:string)  [unwired: 3 in, 1 out]
        n663 = Index Array(array=w1024, index (col) #1=0 ("disabled index (col)"), index (col) #2=1 ("index (col)")) -> (element #1=w1033:string[], element #2=w1031:string[])  [unwired: 2 in]
        n664 = Search 1D Array(1D array=w1033, element=w1032) -> (index of element=w1030:i32)  [unwired: 1 in]
        n665 = disable-structure shown="Disabled" {
          disable-tunnel: w1031 -> [w1073 _]
          disable-tunnel: w1030 -> [w1072 w1074]
          disable-tunnel: w1029 -> [w1071 _]
          disable-tunnel: [w1070 w1074] -> w1023
          frame Disabled {
            n666 = Search 1D Array(1D array=w1073, element=w1071, start index (0)=w1072) -> (index of element=w1070:i32)
          }
          frame Enabled {
          }
        }
        n667 = Index Array(array=w1039, index (col) #1=0 ("disabled index (col)"), index (col) #2=1 ("disabled index (col)")) -> (element #1=w1043:string[], element #2=w1042:string[])  [unwired: 2 in]
        n668 = Format Date/Time String(time format string (%c)="%d%b%y %I:%M:%S %p") -> (date/time string=w1064:string)  [unwired: 2 in]
        n669 = Interleave 1D Arrays(w1043, w1042) -> (w1041:string[])
        n670 = Index Array(array=w1024, index (row)=w1023) -> (element=w1022:string[])  [unwired: 1 in]
        n671 = To Upper Case(1:w1064) -> (0:w1026:string)
        n672 = case shown="False" w1027 {
          tunnel: w1066 -> [w1078 _]
          tunnel: [w1076 w1080] -> w1065
          tunnel: [w1075 w1079] -> w1025
          tunnel: w1026 -> [w1075 _]
          tunnel: w1022 -> [_ w1082]
          frame False {
            n673 = Number To Fractional String(number=w1078, precision (6)=i16 16) -> (F-format string=w1076:string[])  [unwired: 2 in]
          }
          frame True {
            n674 = Array Subset(array=w1082, index=2, length=9) -> (w1080:string[])
            n675 = Index Array(array=w1082, index=11) -> (element=w1079:string)
          }
        }
        n676 = Build Array (concatenate)(w1032, w1029, w1065, w1025, w1041) -> (w1062:string[])
        n677 = Greater?(x=w1023, y=w1053) -> (0:w1052:bool)
        n678 = Subtract(x=w1023, y=w1053) -> (x-y=w1051:i32)
        n679 = Bundle(cluster=T12 {"Row"=0, "Column"=0} ("Active Cell:Active Cell"), "Row"=w1023, "Column"=-2) -> (w1054:T12)
        n680 = Select(t=w1051, s=w1052, f=u16 0 ("y")) -> (s? t:f=w1048:i32)
        n681 = Replace Array Subset(array=w1024, new element=w1062, index (row)=w1023) -> (w1059:string[][])  [unwired: 1 in]
        n682 = Bundle(cluster=T12 {"Row"=0, "Column"=0} ("Active Cell:Active Cell"), "Row"=w1048, "Column"=0) -> (w1047:T12)
        n683 = Build Array (concatenate)(w1060, w1059) -> (w1058:string[][])
        n684 = Insert Into Array(array=w1067, index=0, new element=string[] ["Write to Excel", "Load Cal File", "End Cal", "Increment Channel"]) -> (w1068:string[])
        n685 = property on="Cal Table" class="Tbl (strict)"("Active Cell"=w1054, "Cell BG Color"=u32 16775793, "Index Values"=w1047) -> ()  [unwired: 2 in, 2 out]
        n686 = call-poly <vilib>:"Write To Spreadsheet File.vi"("delimiter (\\t)"="," ("delimiter (\\t)"), "2D data"=w1058, "file path (dialog if empty)"=w1038) -> ()  [unwired: 5 in, 1 out]
      }
      frame "Save Calibration" {
        w1131 = u16 4 ("y")
        n687 = Unbundle By Name(w1106) -> ("Cal File Path"=w1116:path, "Cal Log Header"=w1138:string[], "Cal Log"=w1102:string[][], "Channel to Cal"=w1114:T1, "Cal Unit"=w1115:T2, "Verification"=w1105:bool, "Verify Table"=w1117:string[][])
        n688 = local read "Reading Value 1"() -> (w1099:dbl)
        n689 = local read "Reading Value 2"() -> (w1097:dbl)
        n690 = local read "Reading Value 3"() -> (w1095:dbl)
        n691 = local read "Reading Value 4"() -> (w1093:dbl)
        n692 = local read "Reading Value 5"() -> (w1091:dbl)
        n693 = local read "Cal Value 1"() -> (w1098:dbl)
        n694 = local read "Cal Value 2"() -> (w1096:dbl)
        n695 = local read "Cal Value 3"() -> (w1094:dbl)
        n696 = local read "Cal Value 4"() -> (w1092:dbl)
        n697 = local read "Cal Value 5"() -> (w1090:dbl)
        n698 = local read "a0"() -> (w1089:dbl)
        n699 = local read "a1"() -> (w1088:dbl)
        n700 = local read "a2"() -> (w1087:dbl)
        n701 = local read "a3"() -> (w1086:dbl)
        n702 = local read "a4"() -> (w1085:dbl)
        n703 = Build Array(w1099, w1098, w1097, w1096, w1095, w1094, w1093, w1092, w1091, w1090, w1089, w1088, w1087, w1086, w1085) -> (w1144:dbl[])
        n704 = Format Into String(w1114) -> (resulting string=w1110:string)  [unwired: 3 in, 1 out]
        n705 = Format Into String(w1115) -> (resulting string=w1107:string)  [unwired: 3 in, 1 out]
        n706 = Index Array(array=w1102, index (col) #1=0 ("disabled index (col)"), index (col) #2=1 ("index (col)")) -> (element #1=w1111:string[], element #2=w1109:string[])  [unwired: 2 in]
        n707 = Search 1D Array(1D array=w1111, element=w1110) -> (index of element=w1108:i32)  [unwired: 1 in]
        n708 = disable-structure shown="Enabled" {
          disable-tunnel: w1109 -> [w1151 _]
          disable-tunnel: w1108 -> [w1150 w1152]
          disable-tunnel: w1107 -> [w1149 _]
          disable-tunnel: [w1148 w1152] -> w1101
          frame Disabled {
            n709 = Search 1D Array(1D array=w1151, element=w1149, start index (0)=w1150) -> (index of element=w1148:i32)
          }
          frame Enabled {
          }
        }
        n710 = Index Array(array=w1117, index (col) #1=0 ("disabled index (col)"), index (col) #2=1 ("disabled index (col)")) -> (element #1=w1121:string[], element #2=w1120:string[])  [unwired: 2 in]
        n711 = Format Date/Time String(time format string (%c)="%d%b%y %I:%M:%S %p") -> (date/time string=w1142:string)  [unwired: 2 in]
        n712 = Interleave 1D Arrays(w1121, w1120) -> (w1119:string[])
        n713 = Index Array(array=w1102, index (row)=w1101) -> (element=w1100:string[])  [unwired: 1 in]
        n714 = To Upper Case(1:w1142) -> (0:w1104:string)
        n715 = case shown="False" w1105 {
          tunnel: w1144 -> [w1156 _]
          tunnel: [w1154 w1158] -> w1143
          tunnel: [w1153 w1157] -> w1103
          tunnel: w1104 -> [w1153 _]
          tunnel: w1100 -> [_ w1160]
          frame False {
            n716 = Number To Fractional String(number=w1156, precision (6)=i16 16) -> (F-format string=w1154:string[])  [unwired: 2 in]
          }
          frame True {
            n717 = Array Subset(array=w1160, index=2, length=9) -> (w1158:string[])
            n718 = Index Array(array=w1160, index=11) -> (element=w1157:string)
          }
        }
        n719 = Build Array (concatenate)(w1110, w1107, w1143, w1103, w1119) -> (w1140:string[])
        n720 = Greater?(x=w1101, y=w1131) -> (0:w1130:bool)
        n721 = Subtract(x=w1101, y=w1131) -> (x-y=w1129:i32)
        n722 = Bundle(cluster=T12 {"Row"=0, "Column"=0} ("Active Cell:Active Cell"), "Row"=w1101, "Column"=-2) -> (w1132:T12)
        n723 = Select(t=w1129, s=w1130, f=u16 0 ("y")) -> (s? t:f=w1126:i32)
        n724 = Replace Array Subset(array=w1102, new element=w1140, index (row)=w1101) -> (w1137:string[][])  [unwired: 1 in]
        n725 = Bundle(cluster=T12 {"Row"=0, "Column"=0} ("Active Cell:Active Cell"), "Row"=w1126, "Column"=0) -> (w1125:T12)
        n726 = Build Array (concatenate)(w1138, w1137) -> (w1136:string[][])
        n727 = Insert Into Array(array=w1145, index=0, new element=string[] ["Write to Excel", "Load Cal File", "Cal Review Prep"]) -> (w1146:string[])
        n728 = property on="Cal Table" class="Tbl (strict)"("Active Cell"=w1132, "Cell BG Color"=u32 16775793, "Index Values"=w1125) -> ()  [unwired: 2 in, 2 out]
        n729 = call-poly <vilib>:"Write To Spreadsheet File.vi"("delimiter (\\t)"="," ("delimiter (\\t)"), "2D data"=w1136, "file path (dialog if empty)"=w1116) -> ()  [unwired: 5 in, 1 out]
      }
      frame "Distribute Calibration" {
        # "have to add in waiting screen, reread on main program, switch to streaming calibrated data and verification for that"
        n730 = Unbundle By Name(w1167) -> ("Desired System.ID"=w1164:string, "Cal File Path"=w1169:path)
        n731 = Concatenate Strings("10.30.189." ("string"), w1164) -> (w1165:string)
        n732 = Format Into String(format string="%s.cal", w1164) -> (resulting string=w1166:string)  [unwired: 2 in, 1 out]
        n733 = flat-sequence {
          tunnel: w1165 -> [w1175]
          tunnel: w1166 -> [w1174]
          tunnel: w1169 -> [w1173]
          frame #0 {
            n734 = call <vilib>:"FTP Put File.vi"("password"="", "user"="anonymous", "local path"=w1173, "remote path"=w1174, "host"=w1175) -> ()  [unwired: 5 in, 2 out]
          }
        }
      }
      frame "Calc Dev" {
        n735 = Unbundle By Name(w1183) -> ("Verify Table"=w1180:string[][], "Cal Unit"=w1178:T2, "Rack Version"=w1177:T5, "Verify Table Ref"=w1176:refnum<vi>)
        n736 = call "Calc Dev (DAQ Rack).vi"("Verify Table IN"=w1180, "Units"=w1178, "Rack Version"=w1177, "Dev Table 1 Ref"=w1176) -> ("Verify Table OUT"=w1179:string[][])  [unwired: 15 in]
        n737 = local write "Verify Table"(w1179) -> ()
        n738 = Bundle By Name(cluster=w1183, "Verify Table"=w1179) -> (w1182:T9)
        n739 = Insert Into Array(array=w1185, index=0, new element=string[] []) -> (w1184:string[])
      }
      frame "Write to Excel" {
        n740 = Unbundle By Name(w1194) -> ("Cal Spreadsheet Path"=w1198:path, "Verify Table"=w1191:string[][], "Channel to Cal"=w1188:T1, "Cal Unit"=w1187:T2)
        n741 = flat-sequence {
          tunnel: w1198 -> [w1205]
          tunnel: [w1205] -> w1199
          tunnel: [w1202] -> w1192
          tunnel: w1191 -> [w1202]
          tunnel: [w1201] -> w1190
          tunnel: w1188 -> [w1201]
          tunnel: [w1200] -> w1189
          tunnel: w1187 -> [w1200]
          tunnel: w1199 -> [w1209]
          tunnel: w1192 -> [w1208]
          tunnel: w1190 -> [w1207]
          tunnel: w1189 -> [w1206]
          frame #0 {
            n742 = property on="Main Tab" class="TabCtl (strict)"("DisabledEnum"=T10."Disabled" ("Disabled")) -> ()  [unwired: 2 in, 2 out]
            n743 = property on="Load Indicator Tab" class="TabCtl (strict)"("Visible"=TRUE) -> ()  [unwired: 2 in, 2 out]
          }
          frame #1 {
            n744 = call "New Write DAQ Rack Data.vi"("Cal Unit"=w1206, "Channel to Cal"=w1207, "Verify Table"=w1208, "Cal Path"=w1209) -> ()  [unwired: 8 in]
          }
          frame #2 {
            n745 = property on="Main Tab" class="TabCtl (strict)"("DisabledEnum"=T10."Enabled" ("Disabled")) -> ()  [unwired: 2 in, 2 out]
            n746 = property on="Load Indicator Tab" class="TabCtl (strict)"("Visible"=FALSE) -> ()  [unwired: 2 in, 2 out]
          }
        }
        n747 = Insert Into Array(array=w1196, index=0, new element=string[] ["Recolor Tables"]) -> (w1195:string[])
      }
      frame "Recolor Tables" {
        n748 = Unbundle By Name(w1216) -> ("Verify Table Ref"=w1215:refnum<vi>)
        n749 = property on="Property Node" class="Tbl (strict)"(reference=w1215, "Active Cell"=T12 {"Row"=-2, "Column"=-2} ("Active Cell:Active Cell"), "Cell BG Color"=u32 15527148) -> (reference out=w1212:refnum<vi>)  [unwired: 1 in, 1 out]
        n750 = property on="Property Node" class="Tbl (strict)"(reference=w1212, "Active Cell"=T12 {"Row"=-2, "Column"=1} ("Active Cell:Active Cell"), "Cell BG Color"=u32 16448250) -> ()  [unwired: 1 in, 2 out]
      }
      frame "End Cal" {
        w1220 = FALSE ("1st Point Cal")
        w1222 = T10."Disabled and Grayed Out" ("Disabled")
        w1224 = 0.0 ("Reading Value 1")
        w1228 = FALSE ("Visible")
        n751 = disable-structure shown="Disabled" {
          frame Disabled {
            n752 = property on="Cancel Verify" class="Bool"("Value"=FALSE ("Cancel Cal")) -> ()  [unwired: 2 in, 2 out]
          }
          frame Enabled {
          }
        }
        n753 = property on="Output Tab" class="TabCtl (strict)"("Visible"=w1228) -> ()  [unwired: 2 in, 2 out]
        n754 = property on="Header Tab" class="TabCtl (strict)"("Visible"=w1228) -> ()  [unwired: 2 in, 2 out]
        n755 = property on="Load Indicator Tab" class="TabCtl (strict)"("Visible"=w1228) -> ()  [unwired: 2 in, 2 out]
        n756 = property on="Main Tab" class="TabCtl (strict)"("DisabledEnum"=T10."Enabled" ("Disabled")) -> ()  [unwired: 2 in, 2 out]
        n757 = property on="Header" class="Bool"("DisabledEnum"=T10."Enabled" ("Disabled")) -> ()  [unwired: 2 in, 2 out]
        n758 = local write "Reading Value 1"(w1224) -> ()
        n759 = local write "Cal Value 1"(w1224) -> ()
        n760 = local write "Reading Value 2"(w1224) -> ()
        n761 = local write "Cal Value 2"(w1224) -> ()
        n762 = local write "Reading Value 3"(w1224) -> ()
        n763 = local write "Cal Value 3"(w1224) -> ()
        n764 = local write "Reading Value 4"(w1224) -> ()
        n765 = local write "Cal Value 4"(w1224) -> ()
        n766 = local write "Reading Value 5"(w1224) -> ()
        n767 = local write "Cal Value 5"(w1224) -> ()
        n768 = local write "a0"(w1224) -> ()
        n769 = local write "a1"(w1224) -> ()
        n770 = local write "a2"(w1224) -> ()
        n771 = local write "a3"(w1224) -> ()
        n772 = local write "a4"(w1224) -> ()
        n773 = property on="Start Cal" class="Bool"("DisabledEnum"=w1222) -> ()  [unwired: 2 in, 2 out]
        n774 = property on="Channel to Cal" class="Enum (strict)"("DisabledEnum"=w1222) -> ()  [unwired: 2 in, 2 out]
        n775 = property on="View Spreadsheet" class="Bool"("DisabledEnum"=w1222) -> ()  [unwired: 2 in, 2 out]
        n776 = property on="Start Verification" class="Bool"("DisabledEnum"=w1222) -> ()  [unwired: 2 in, 2 out]
        n777 = local write "RIO Found"(FALSE ("RIO Found")) -> ()
        n778 = local write "Tank IP:"("" ("Tank IP:")) -> ()
        n779 = call "TCP Data Stream PC.vi"("Mode"=TCP_Data_Stream_Mode_(PC)."Close") -> ()  [unwired: 15 in, 4 out]
        n780 = disable-structure shown="Disabled" {
          disable-tunnel: w1222 -> [w1234 _]
          frame Disabled {
            n781 = property on="Cal Unit" class="Enum (strict)"("DisabledEnum"=w1234) -> ()  [unwired: 2 in, 2 out]
          }
          frame Enabled {
          }
        }
        n782 = local write "1st Point Cal"(w1220) -> ()
        n783 = local write "2nd Point Cal"(w1220) -> ()
        n784 = local write "3rd Point Cal"(w1220) -> ()
        n785 = local write "4th Point Cal"(w1220) -> ()
        n786 = local write "5th Point Cal"(w1220) -> ()
        n787 = Insert Into Array(array=w1232, index=0, new element=string[] ["Recolor Tables", "Init Cal"]) -> (w1233:string[])
      }
      frame "Increment Channel" {
        n788 = Unbundle By Name(w1238) -> ("Channel to Cal"=w1237:T1)
        n789 = Increment(x=w1237) -> (x+1=w1236:T1)
        n790 = Bundle By Name(cluster=w1238, "Channel to Cal"=w1236) -> (w1239:T9)
        n791 = local write "Channel to Cal"(w1236) -> ()
      }
      frame "Exit" {
        n792 = local write "Stop Second Loop"(TRUE ("Stop Second Loop")) -> ()
      }
    }
  }
  n793 = while {
    tunnel: w1 -> [_]
    shift-right: [w1244] -> _
    shift-left: _ -> [w1245]
    stop <- "Stop Second Loop" stop-if-true
    n794 = local read "Channel to Cal"() -> (w1248:T1)
    n795 = local read "RIO Found"() -> (w1249:bool)
    n796 = Wait (ms)(milliseconds to wait=u32 10) -> ()  [unwired: 1 out]
    n797 = case shown="True" w1249 {
      tunnel: w1248 -> [_ w1255]
      tunnel: [0.0 ("Data Out") w1253] -> w1244
      tunnel: w1245 -> [_ w1252]
      frame False {
        n798 = Wait (ms)(milliseconds to wait=u32 500) -> ()  [unwired: 1 out]
      }
      frame True {
        n799 = call "New DAQ Rack AI Read.vi"("Channel to Cal"=w1255) -> ("Lost Connection"=→"Lost Connection":bool, "Available?"=w1257:bool, "Data"=w1256:dbl)  [unwired: 8 in]
        n800 = case shown="True" w1257 {
          tunnel: w1256 -> [_ w1263]
          tunnel: w1255 -> [_ w1262]
          tunnel: [w1258 w1260] -> w1253
          tunnel: w1252 -> [w1258 _]
          frame False {
          }
          frame True {
            n801 = call <vilib>:"Mean PtByPt.vi"("x"=w1263, "sample length"="avg") -> ("mean"=w1261:dbl)  [unwired: 2 in, 1 out]
            n802 = local read "Cal Unit"() -> (w1259:T2)
            n803 = call "D2A_5V.vi"("Channel to Cal"=w1262, "Data In"=w1261, "Cal Unit"=w1259) -> ("Data Out"=w1260:dbl)  [unwired: 12 in]
          }
        }
      }
    }
    "Cal Reading" <- w1244
    "Ver Reading" <- w1244
  }
  n804 = disable-structure shown="Disabled" {
    frame Disabled {
      n805 = property on="Verify Tab" class="TabCtl (strict)"("Visible"=TRUE) -> (error out=w1266:errorcluster)  [unwired: 2 in, 1 out]
      n806 = property on="Verify Table" class="Tbl (strict)"(error in=w1266, "Key Focus"=TRUE, "EditPos"=T12 {"Row"=0, "Column"=1} ("Active Cell:Active Cell")) -> ()  [unwired: 1 in, 2 out]
    }
    frame Enabled {
    }
  }
  n807 = disable-structure shown="Disabled" {
    frame Disabled {
      w1290 = 0 ("length")
      # "#Change In \"A\" selection added selection of \"RIO\" that links 25A Targets and Setpoints"
      n808 = Unbundle By Name() -> (w1286:T16, "Cal Targets Path"=w1279, "Targets"=w1284, "Cal Target Array"=w1300, "Channel to Cal"=w1301, "Verify Table"=w1273)
      n809 = property on="Cancel Verify" class="Bool"("DisabledEnum"=T10."Enabled" ("Disabled")) -> ()  [unwired: 2 in, 2 out]
      n810 = property on="Cal Table" class="Tbl (strict)"("Active Cell"=T12 {"Row"=-2, "Column"=-2} ("Active Cell:Active Cell"), "Cell BG Color"=u32 16448250) -> ()  [unwired: 2 in, 2 out]
      n811 = call <vilib>:"Open Config Data.vi"("configuration file path"=w1279) -> ("error out"=w1281:errorcluster, "refnum"=w1280:T15)  [unwired: 8 in, 1 out]
      n812 = call <userlib>:"Read INI Cluster__ogtk.vi"("error in (no error)"=w1281, "INI Fomatted Cluster Type"=w1284, "refnum"=w1280) -> ("error out"=w1283:errorcluster, "INI Fomatted Cluster"=w1285:variant, "dup refnum"=w1282:T15)  [unwired: 4 in, 2 out]
      n813 = Index Array(array=w1300, index=w1301) -> (element=w1296)
      n814 = call <vilib>:"Close Config Data.vi"("error in (no error)"=w1283, "refnum"=w1282) -> ()  [unwired: 8 in, 2 out]
      n815 = Variant To Data(type=w1284, Variant=w1285) -> (data=w1297)  [unwired: 1 in, 1 out]
      n816 = case shown="\"V\", Default" w1296 {
        tunnel: w1297 -> [w1306 w1309 w1312 w1315 w1318 w1321]
        tunnel: [w1304 w1307 w1310 w1313 w1316 w1319] -> w1299
        tunnel: [w1305 w1308 w1311 w1314 w1317 w1320] -> w1298
        frame "V", Default {
          n817 = Unbundle By Name(w1306) -> ("V Targets"=w1305, "V Setpoints"=w1304)
        }
        frame "A" {
          n818 = Unbundle By Name(w1309) -> ("A Targets"=w1308, "A Setpoints"=w1307)
        }
        frame "DegC" {
          n819 = Unbundle By Name(w1312) -> ("DegC Targets"=w1311, "DegC Setpoints"=w1310)
        }
        frame "kPa" {
          n820 = Unbundle By Name(w1315) -> ("kPa Targets"=w1314, "kPa Setpoints"=w1313)
        }
        frame "LpH" {
          n821 = Unbundle By Name(w1318) -> ("LpH Targets"=w1317, "LpH Setpoints"=w1316)
        }
        frame "CT" {
          n822 = Unbundle By Name(w1321) -> ("CT Targets"=w1320, "CT Setpoints"=w1319)
        }
      }
      n823 = Cluster To Array(cluster=w1298) -> (array=w1289:void[])
      n824 = Cluster To Array(cluster=w1299) -> (array=w1288:void[])
      n825 = Delete From Array(array=w1289, length=w1290, index=w1290) -> (deleted portion=w1294, array with subset deleted=w1291)
      n826 = call-poly <userlib>:"Remove Duplicates from 1D Array__ogtk.vi"("Input Array"=w1291) -> ("Output Array"=w1292:dbl[])  [unwired: 1 out]
      n827 = Build Array (concatenate)(w1294, w1292) -> (w1293:dbl[])
      n828 = Number To Fractional String(number=w1293, precision (6)=i16 3) -> (F-format string=w1287:string[])  [unwired: 2 in]
      n829 = Index Array(array=w1288) -> (element #1=w1276, element #2=w1277, element #3=w1278, element #4=w1302, element #5=w1303)  [unwired: 5 in]
      n830 = Replace Array Subset(array=w1273, new element=w1287, index (col)=0 ("disabled index (col)")) -> (w1275:string[])  [unwired: 1 in]
      n831 = local write "Cal Value 1"(w1276) -> ()
      n832 = local write "Cal Value 2"(w1277) -> ()
      n833 = local write "Cal Value 3"(w1278) -> ()
      n834 = local write "Cal Value 4"(w1302) -> ()
      n835 = local write "Cal Value 5"(w1303) -> ()
      n836 = Bundle By Name(cluster=w1286, "Targets"=w1297, "Verify Table"=w1275) -> (w1272:cluster{})
      n837 = property on="Verify Table" class="Tbl (strict)"("Value"=w1275) -> ()  [unwired: 2 in, 2 out]
    }
    frame Enabled {
    }
  }
